vi "pyonpyon3.vi"() -> ()   [LabVIEW 2013]
uses:
  impl/pp3_CTL_SessionInfo.ctl
  impl/pp3_CTL_StateInfo.ctl
  impl/pp3_CTL_State.ctl
  impl/pp3_CTL_Trial.ctl
  impl/pp3_CTL_TrialType.ctl
  labolabo2/waveforms/WFTypes.ctl
  impl/pp2_CTL_SessionParamDynamic.ctl
  impl/pp2_CTL_DaqConfig.ctl
  <vilib>/userdefined/High Color/IMAQdx.ctl
  <vilib>/sound2/lvsound2.llb/Sound Output Task ID.ctl
  labolabo2/array/impl/NullArray_I.vi
  <vilib>/Utility/file.llb/Read From Spreadsheet File (string).vi
  labolabo2/array/impl/ArrayFirst_S.vi
panel:
  in  "Session List Hidden":u8[](array[numeric]) min=1 step=1
  out "concatenated string":string="OS Name:                   Microsoft Wi\rOS Version:                6.1.7601 Service Pack 1 Build 7601\rSystem Type:               x64-based PC\rTime Zone:                 (UTC+01:00) Amsterdam, Berli\rTotal Physical Memory:     7,657 MB"
  out "Info VI Revision":string="1221" caption="Rev #"
  out "Info VI Name":string="pyonpyon2.vi"
  out "Info Hostname":string="PCR6985-17"
  out "Session list display":string[][](table)
  in  "Trial Types Control":enum32{"Trial Types Control"}(tab)
  out "Trial Types File Path":path=path "E:/Data/SPP.Coulb1/trial types/FM2k4k_4k2k.pp2tt.tsv"
  in  "Save Trial Types":bool
  in  "Load Trial Types":bool
  out "Trial Types Valid":bool
  in  "Trial Types":T1[](array[typedef])=[{"Trial Type Number"=1, "Trial Type"=enum."GO", "Trial Weight"=1, "Shock (mA)"=-1.0, "Duration (ms)"=250.0, "Sound Type"=enum."04 FM Sweep", "Stim P1"=2000.0, "Stim P2"=4000.0, "Stim P3"=0.0, "Stim P4"=0.0, "DAQ Amplitude (V)"=0.25}, {"Trial Type Number"=2, "Trial Type"=enum."NOGO", "Trial Weight"=1, "Shock (mA)"=-1.0, "Duration (ms)"=250.0, "Sound Type"=enum."04 FM Sweep", "Stim P1"=4000.0, "Stim P2"=2000.0, "Stim P3"=0.0, "Stim P4"=0.0, "DAQ Amplitude (V)"=0.25}] {"DAQ Amplitude (V)" min=0.0 max=5.0 format="%_6g"; "Shock (mA)" min=-1.0 max=5.0; "Trial Weight" step=1; "Duration (ms)" min=0.0 max=1.0; "Trial Type Number" min=1 max=256 step=1}
  in  "Session List Control":enum32{"Session List Control"}(tab)
  out "Session List File Path":path
  in  "Load Session List":bool
  in  "Save Session List":bool
  in  "Generate Session List":bool
  in  "Total Trials":i32=60 min=3 max=122 step=1
  in  "Pseudo-Gellerman\nStart":i32=2 min=0 max=3 step=1
  out "Session List Valid":bool
  in  "Daq config":T4={"Sound AO"="Dev3/ao0", "Shock intesity AO"="Dev3/ao1", "Code_LED DO"="Dev3/port0", "Switch DI"="Dev3/port2/line0", "Webcam"="cam9", "Sound AO task"="", "Sound card task"=0, "Shock intensity AO task"="", "Code_LED DO task"="", "Switch DI task"="", "AO <=> Sound card"=FALSE, "Sound card"=0, "sample rate"=100000.0, "Variable shock"=TRUE, "Webcam on"=TRUE, "Tone gate PFI"="/Dev3/PFI0", "Waveform memo"={"t0"=timestamp(0 s since 1904-01-01), "dt"=1.0, "Y"=[]}, "First time"=FALSE} {"sample rate" min=8000.0; "Sound card task" format="%.0x"}
  out "Image":T7(plugin-control)
  in  "Session param (dynamic)":T8={"Def M shock (mA)"=700.0, "Def F shock (mA)"=140.0, "Def M shock +/-"=4, "Def F shock +/-"=4} {"Def F shock +/-" min=0 step=1; "Def M shock +/-" min=0 step=1}
  in  "stop":bool
  in  "Pause":bool
  out "State info":T9={"Curr  tr"=6, "Curr (ms)"=314431, "Cum (ms)"=205111, "Run loop diff"=6, "Tone countdown (ms)"=999999, "Countdown (ms)"=-1, "Curr State"=enum."15 Done", "Prev State"=enum."14 Intertrial Interval", "Rw"=FALSE, "Sw"=TRUE, "Tone\nGate"=FALSE, "Punish"=FALSE, "Current DAQ DO Int"=0, "Current Loaded Trial"={"Trial Type Number"=2, "Trial Type"=enum."NOGO", "Trial Weight"=1, "Shock (mA)"=0.0, "Duration (ms)"=250.0, "Sound Type"=enum."04 FM Sweep", "Stim P1"=4000.0, "Stim P2"=2000.0, "Stim P3"=0.0, "Stim P4"=0.0, "DAQ Amplitude (V)"=0.25}, "Next Trial (for display purposes)"={"Trial Type Number"=1, "Trial Type"=enum."GO", "Trial Weight"=1, "Shock (mA)"=-1.0, "Duration (ms)"=250.0, "Sound Type"=enum."04 FM Sweep", "Stim P1"=2000.0, "Stim P2"=4000.0, "Stim P3"=0.0, "Stim P4"=0.0, "DAQ Amplitude (V)"=0.25}, "Total trials memo"=6, "State start cum memo (ms)"=190105, "Last dur jump time memo (ms)"=0, "Last dur shock time memo (ms)"=0, "Tone repeat memo (ms)"=0, "Webcam on"=TRUE, "Webcam recording"=FALSE, "State update flag"=FALSE, "Last loaded shock voltage"=0.0, "Vid upd"=enum."0"} {"Current DAQ DO Int" format="%016b"; "Next Trial (for display purposes)"."DAQ Amplitude (V)" min=0.0 max=5.0 format="%_6g"; "Next Trial (for display purposes)"."Shock (mA)" min=-1.0 max=5.0; "Next Trial (for display purposes)"."Trial Weight" step=1; "Next Trial (for display purposes)"."Duration (ms)" min=0.0 max=1.0; "Next Trial (for display purposes)"."Trial Type Number" min=1 max=256 step=1; "Current Loaded Trial"."DAQ Amplitude (V)" min=0.0 max=5.0 format="%_6g"; "Current Loaded Trial"."Shock (mA)" min=-1.0 max=5.0; "Current Loaded Trial"."Trial Weight" step=1; "Current Loaded Trial"."Duration (ms)" min=0.0 max=1.0; "Current Loaded Trial"."Trial Type Number" min=1 max=256 step=1}
  in  "Session parameters":T11={"Log File Directory Root"=path "E:/Data/SPP.Coulb1", "Habit tr0 (s)"=180, "ITI max\n(s)"=24, "ITI min\n(s)"=14, "Tone repeat (ms)"=0, "Jump time\n(s)"=4, "Subject Name"="SPP046", "Run"=FALSE, "Start trial"=0, "Stay \n(s)"=5, "Log File Directory"=path "E:/Data/SPP.Coulb1/Test/150117/130444", "Shock \ndur (s)"=6, "Pre click \n(V)"=0.1, "Click\ndel (s)"=1.0, "Reward CR"=FALSE} {"Click\ndel (s)" min=0.0 step=1.0; "Pre click \n(V)" min=0.0 max=1.0 step=1.0; "Shock \ndur (s)" min=0 step=1; "Stay \n(s)" min=0 step=1; "Start trial" step=1; "Jump time\n(s)" min=0 step=1; "Tone repeat (ms)" min=0 max=1000 step=1; "ITI min\n(s)" min=0 step=1; "ITI max\n(s)" min=0 step=1; "Habit tr0 (s)" min=0 step=1}
  out "Runtime Errors":errorcluster
  in  "Refresh":bool
  out "Session info":T12={"Total  Tr"=6, "G Tr"=3, "G Jump"=0, "G Jump%"=0.0, "N Tr"=3, "N Jump"=0, "N Jump%"=0.0, "T Tr"=0, "T Jump"=0, "T Jump%"=nan, "M shock dur (ms)"=59414.666666666664, "F shock dur (ms)"=0.0, "H latency (ms)"=0.0, "F latency (ms)"=0.0, "T jump latency (ms)"=0.0} {"T Jump%" format="%.3g"; "N Jump%" format="%.3g"; "G Jump%" format="%.3g"}
  # "Pyonpyon Labview  v3 \n(2015.10 KT)"
  # "Code"
  # "Type"
  # "Dur (ms)"
  # "P 1"
  # "P 2"
  # "P 3"
  # "P 4"
  # "Weight"
  # "Shock"
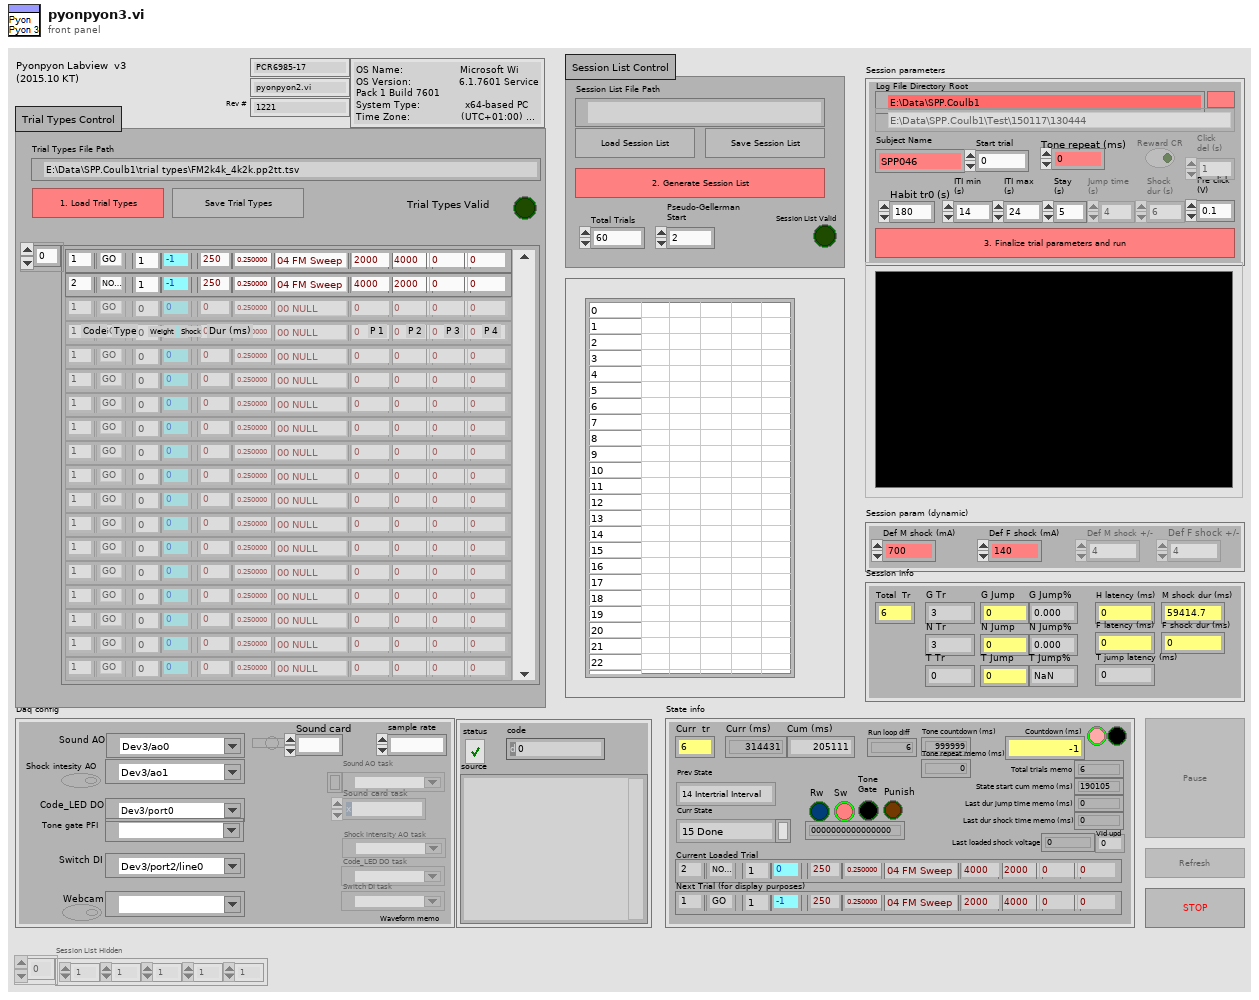
[diagram p1: front panel]
types:
  T1 = typedef "pp3_CTL_Trial.ctl" = cluster{"Trial Type Number":i16, "Trial Type":T2, "Trial Weight":u32, "Shock (mA)":dbl, "Duration (ms)":dbl, "Sound Type":T3, "Stim P1":dbl, "Stim P2":dbl, "Stim P3":dbl, "Stim P4":dbl, "DAQ Amplitude (V)":dbl}
  T2 = typedef "pp3_CTL_TrialType.ctl" = enum16{"OFF", "GO", "NOGO", "TEST"}
  T3 = typedef "WFTypes.ctl" = enum16{"00 NULL", "01 DC", "02 Noise", "03 Pure Tone", "04 FM Sweep"}
  T4 = typedef "pp2_CTL_DaqConfig.ctl" = cluster{"Sound AO":tag, "Shock intesity AO":tag, "Code_LED DO":tag, "Switch DI":tag, "Webcam":T5, "Sound AO task":refnum<k21>, "Sound card task":T6, "Shock intensity AO task":refnum<k21>, "Code_LED DO task":refnum<k21>, "Switch DI task":refnum<k21>, "AO <=> Sound card":bool, "Sound card":u32, "sample rate":dbl, "Variable shock":bool, "Webcam on":bool, "Tone gate PFI":tag, "Waveform memo":waveform(dbl), "First time":bool}
  T5 = typedef "IMAQdx.ctl" = refnum<k21>
  T6 = typedef "Sound Output Task ID.ctl" = u32
  T7 = typedef "IMAQ Image.ctl" = refnum<image>
  T8 = typedef "pp2_CTL_SessionParamDynamic.ctl" = cluster{"Def M shock (mA)":dbl, "Def F shock (mA)":dbl, "Def M shock +/-":i32, "Def F shock +/-":i32}
  T9 = typedef "pp3_CTL_StateInfo.ctl" = cluster{"Curr  tr":u16, "Curr (ms)":u32, "Cum (ms)":i64, "Run loop diff":i64, "Tone countdown (ms)":i64, "Countdown (ms)":i64, "Curr State":T10, "Prev State":T10, "Rw":bool, "Sw":bool, "Tone\nGate":bool, "Punish":bool, "Current DAQ DO Int":u16, "Current Loaded Trial":T1, "Next Trial (for display purposes)":T1, "Total trials memo":i64, "State start cum memo (ms)":i64, "Last dur jump time memo (ms)":i64, "Last dur shock time memo (ms)":i64, "Tone repeat memo (ms)":i64, "Webcam on":bool, "Webcam recording":bool, "State update flag":bool, "Last loaded shock voltage":dbl, "Vid upd":enum16{"0", "1", "2", "3", "4", "5", "6", "7", "8", "9"}}
  T10 = typedef "pp3_CTL_State.ctl" = enum8{"0 NULL", "1 Habituation", "2 (Load Trial)", "3 Stay Period", "4 Load Audio/Click Delay", "5 GO Trial", "6 GO Jumped", "7 GO Timeout", "8 NOGO Trial", "9 NOGO Jumped", "10 NOGO Timeout", "11 TEST Trial", "12 TEST Jumped", "13 TEST Timeout", "14 Intertrial Interval", "15 Done"}
  T11 = cluster{"Log File Directory Root":path, "Habit tr0 (s)":i32, "ITI max\n(s)":i32, "ITI min\n(s)":i32, "Tone repeat (ms)":i32, "Jump time\n(s)":i32, "Subject Name":string, "Run":bool, "Start trial":u16, "Stay \n(s)":i32, "Log File Directory":path, "Shock \ndur (s)":i32, "Pre click \n(V)":dbl, "Click\ndel (s)":dbl, "Reward CR":bool}
  T12 = typedef "pp3_CTL_SessionInfo.ctl" = cluster{"Total  Tr":u32, "G Tr":u32, "G Jump":u32, "G Jump%":dbl, "N Tr":u32, "N Jump":u32, "N Jump%":dbl, "T Tr":u32, "T Jump":u32, "T Jump%":dbl, "M shock dur (ms)":dbl, "F shock dur (ms)":dbl, "H latency (ms)":dbl, "F latency (ms)":dbl, "T jump latency (ms)":dbl}
  T13 = enum8{"Enabled", "Disabled", "Disabled and Grayed Out"}
  T14 = enum16{"open", "replace", "create", "open or create", "replace or create", "replace or create with confirmation"}
  T15 = typedef "imagedata.ctl" = cluster{"image type":i32, "image depth":i32, "image":u8[], "mask":u8[], "colors":u32[], "Rectangle":cluster{"left":i16, "top":i16, "right":i16, "bottom":i16}}
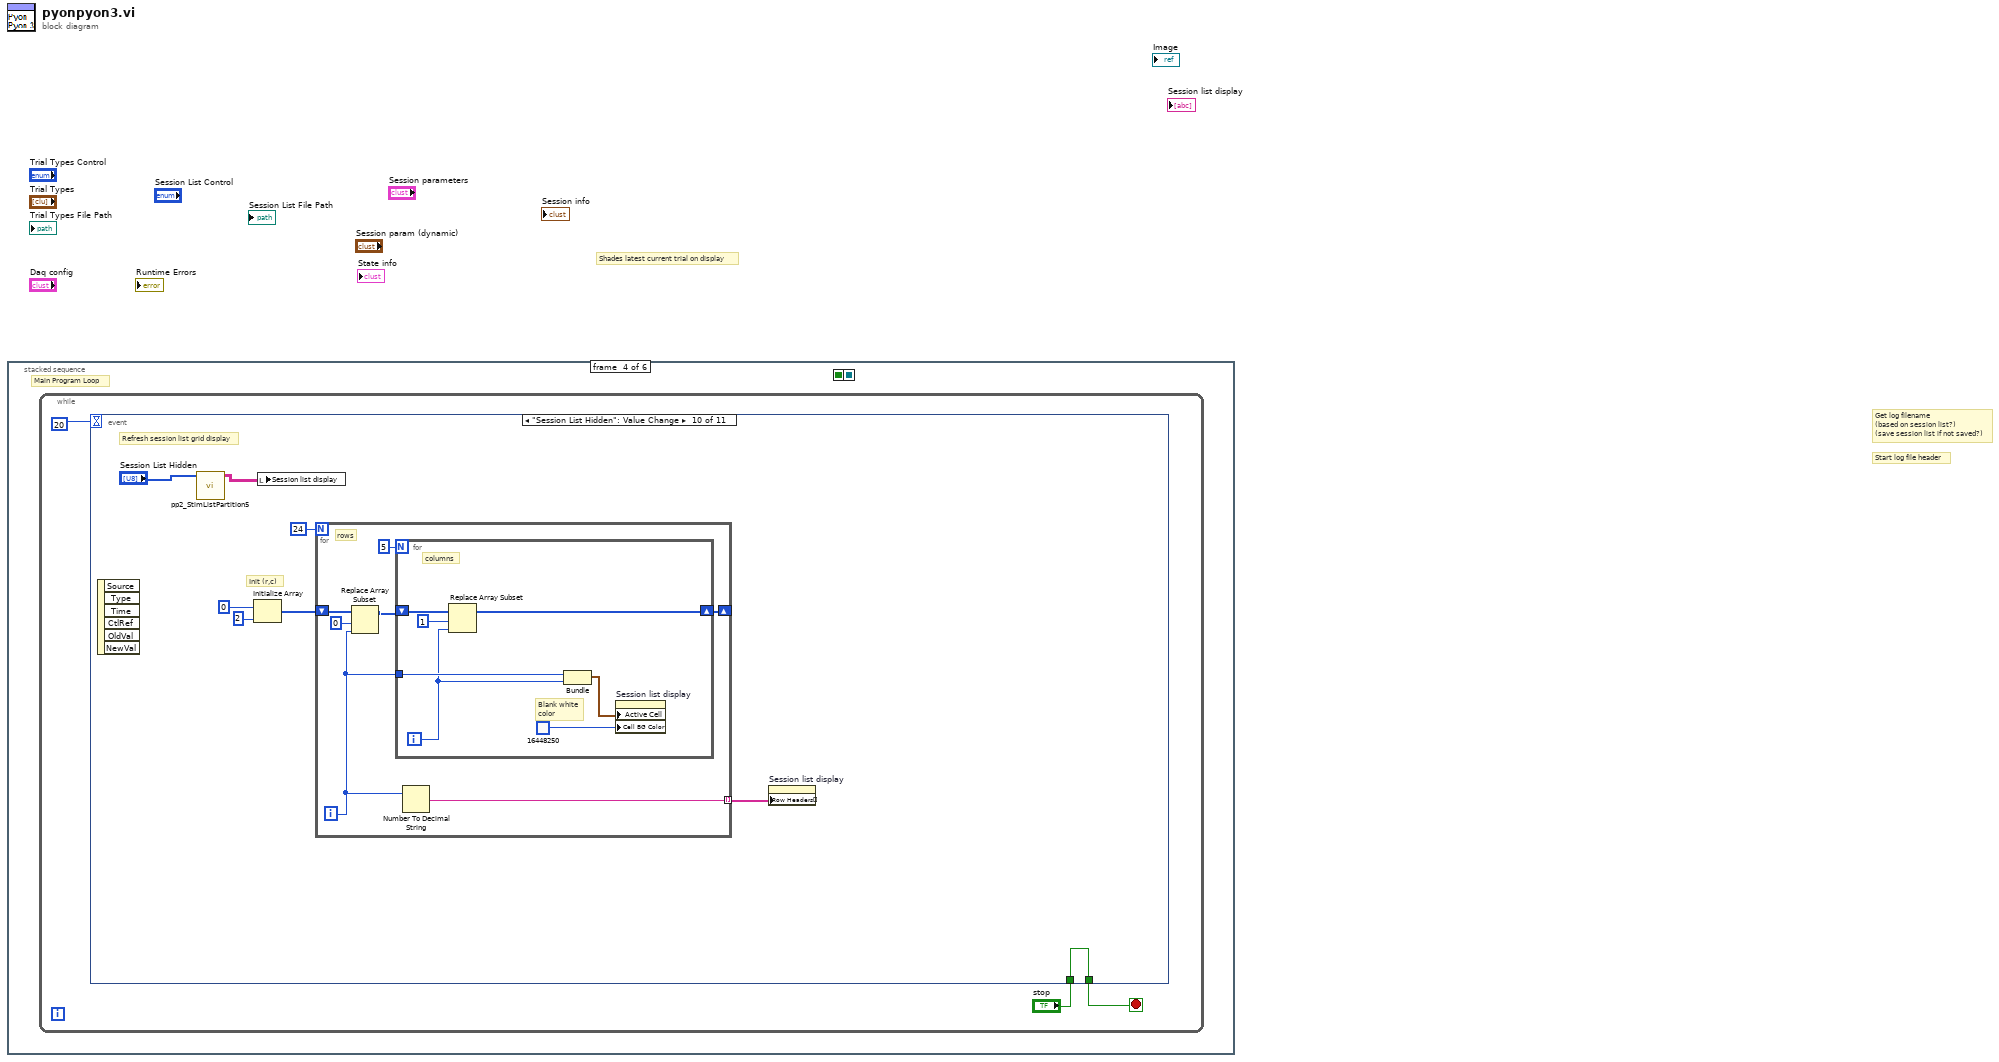
[diagram p0: block diagram]
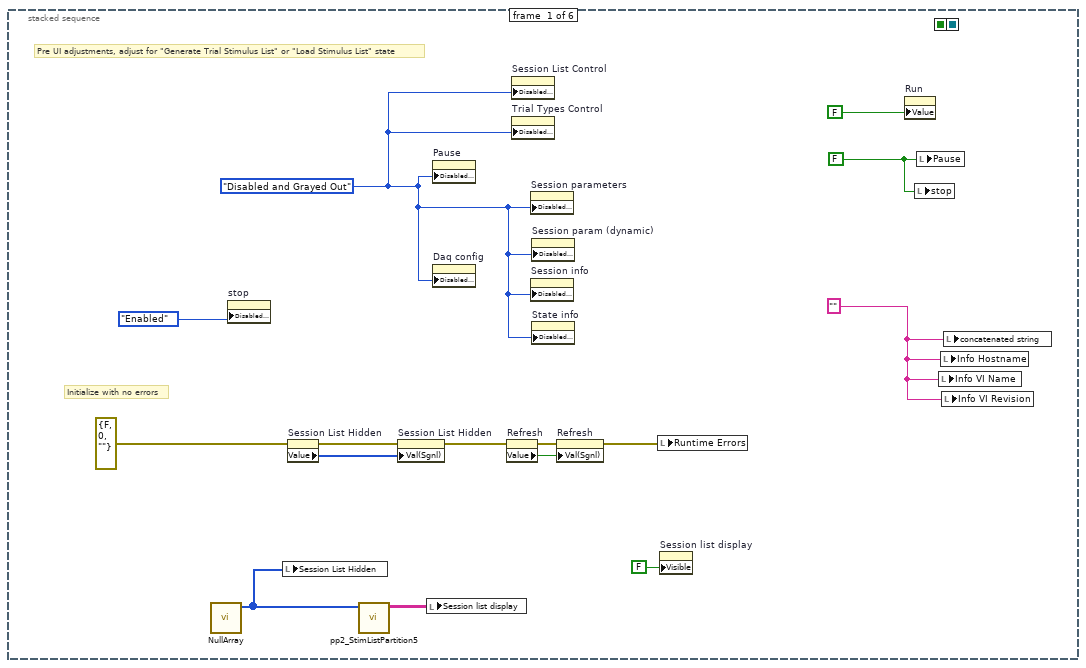
[diagram p2: hidden frame]
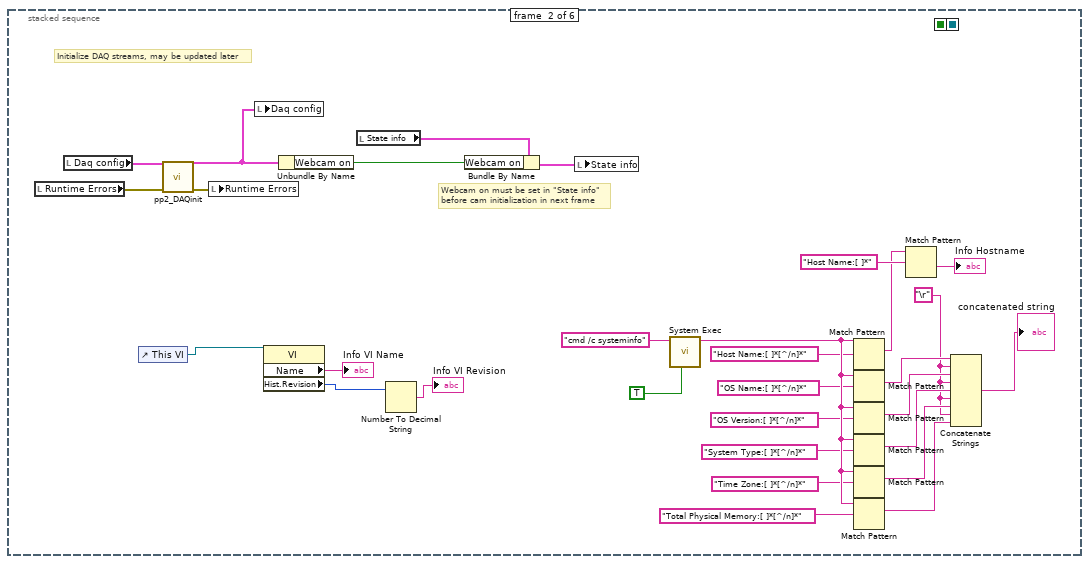
[diagram p3: hidden frame]
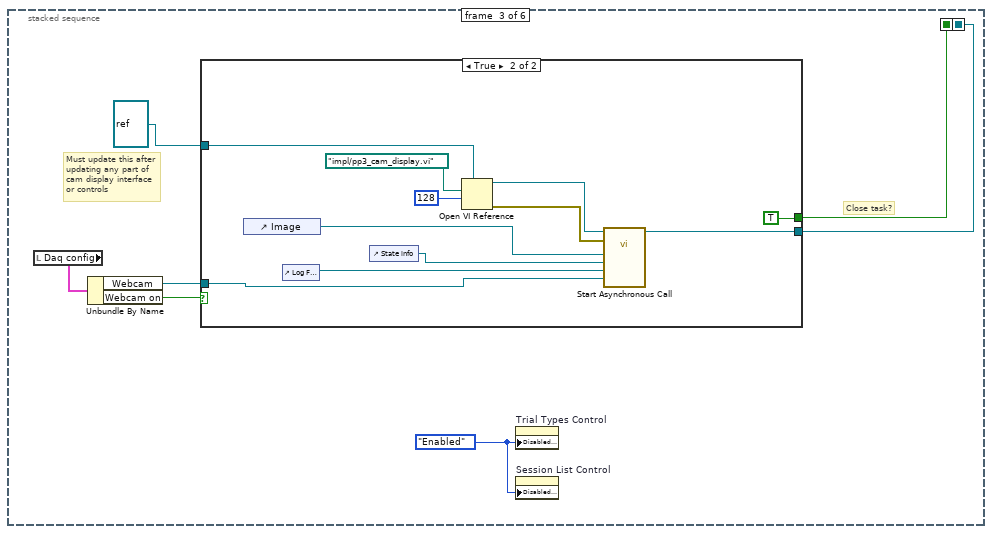
[diagram p4: hidden frame]
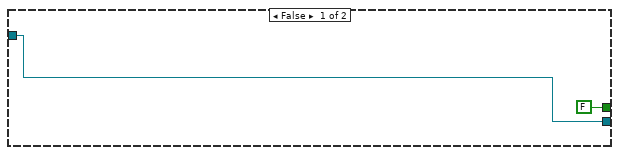
[diagram p5: hidden frame]
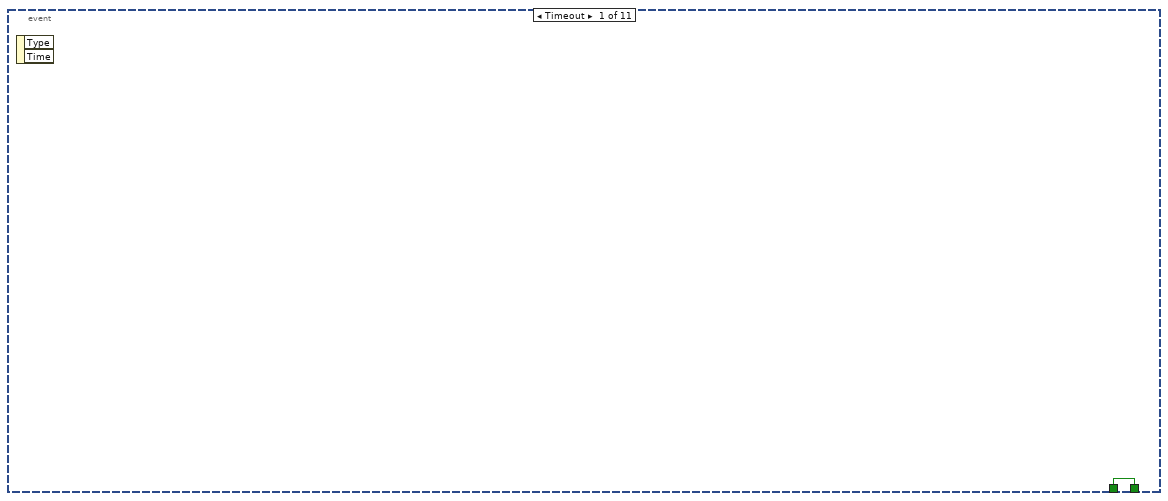
[diagram p6: hidden frame]
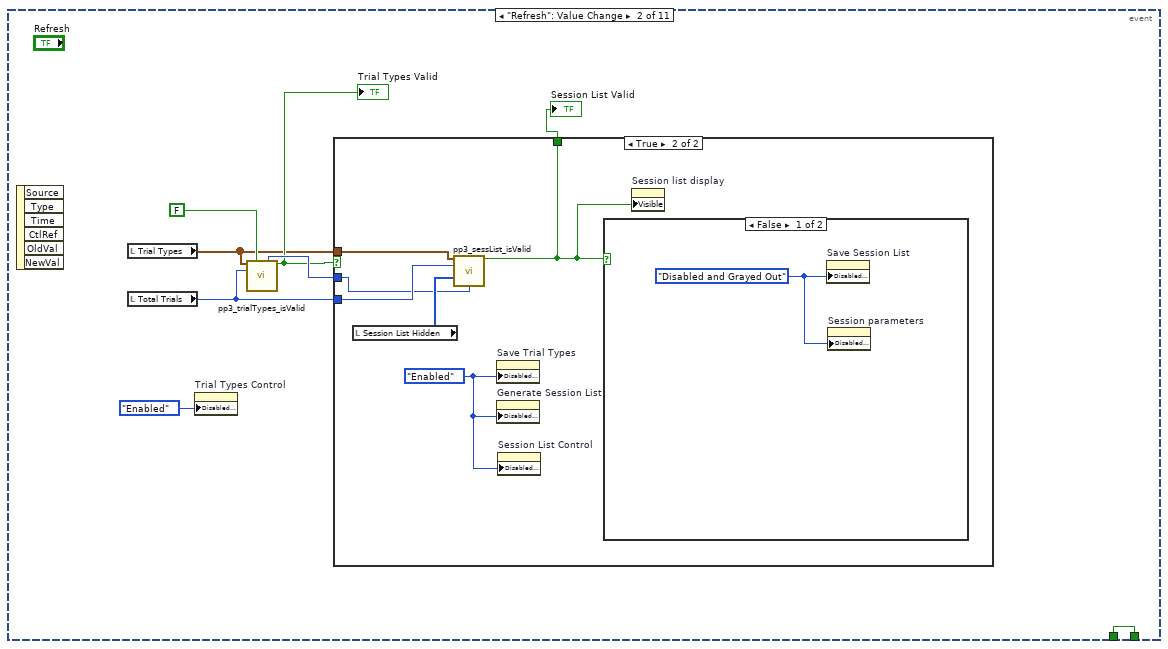
[diagram p7: hidden frame]
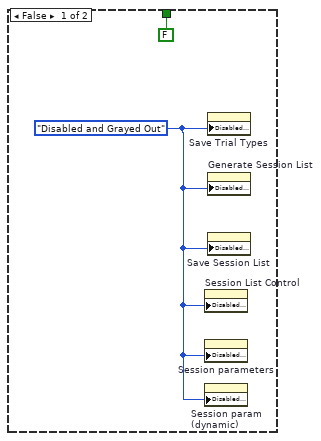
[diagram p8: hidden frame]
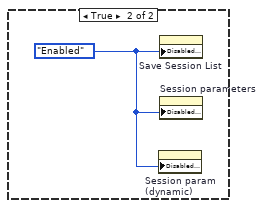
[diagram p9: hidden frame]
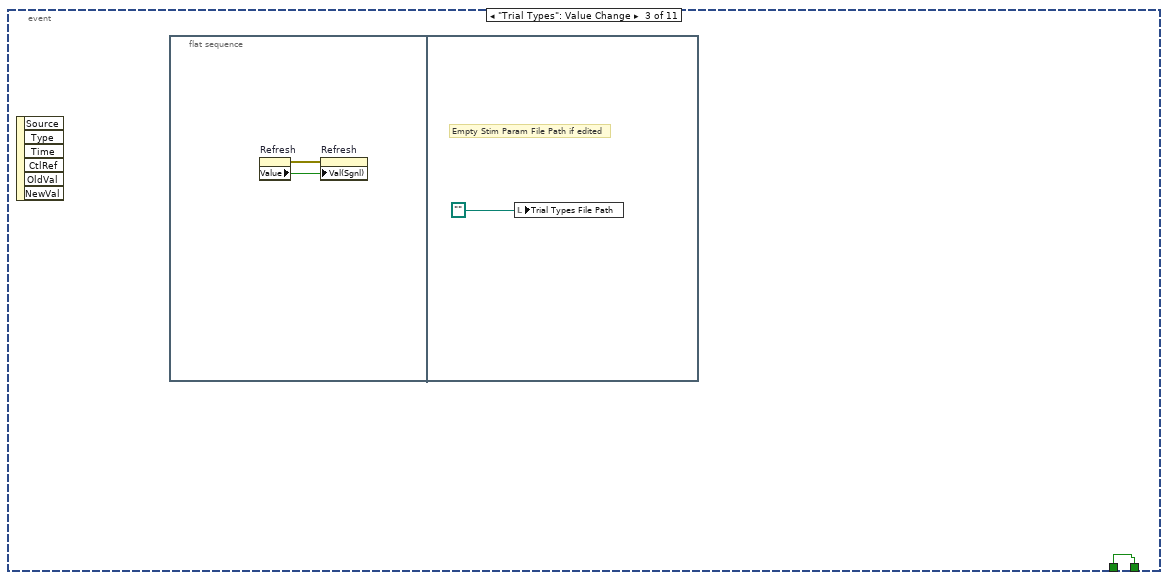
[diagram p10: hidden frame]
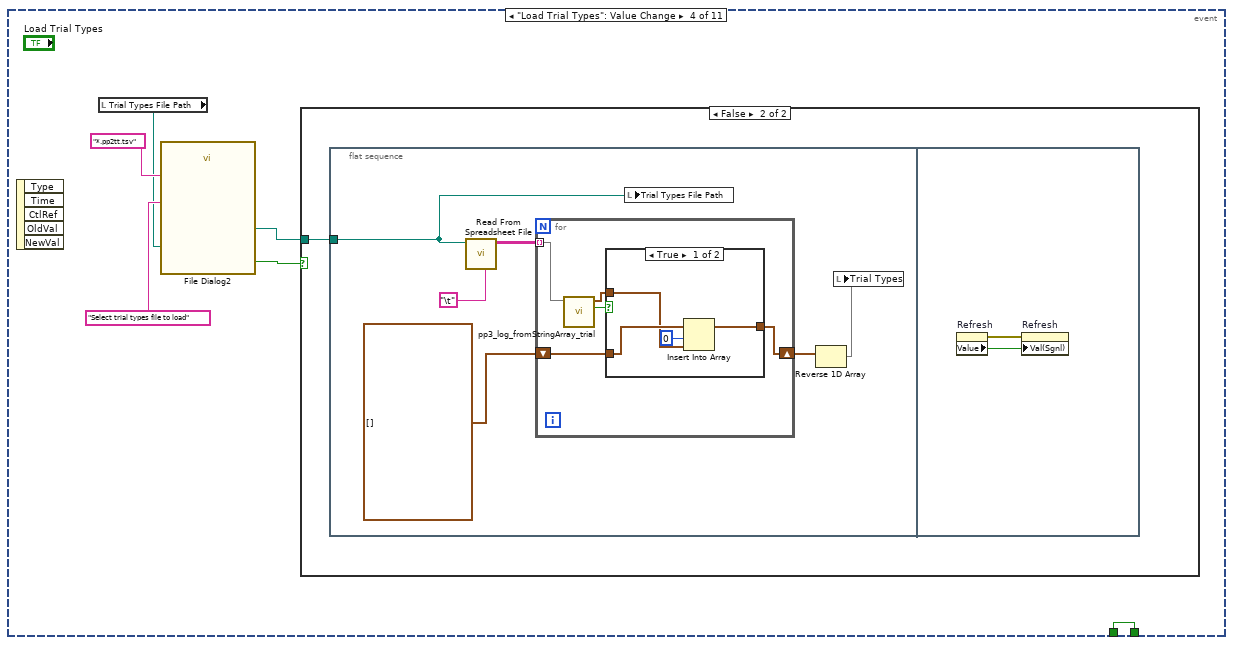
[diagram p11: hidden frame]
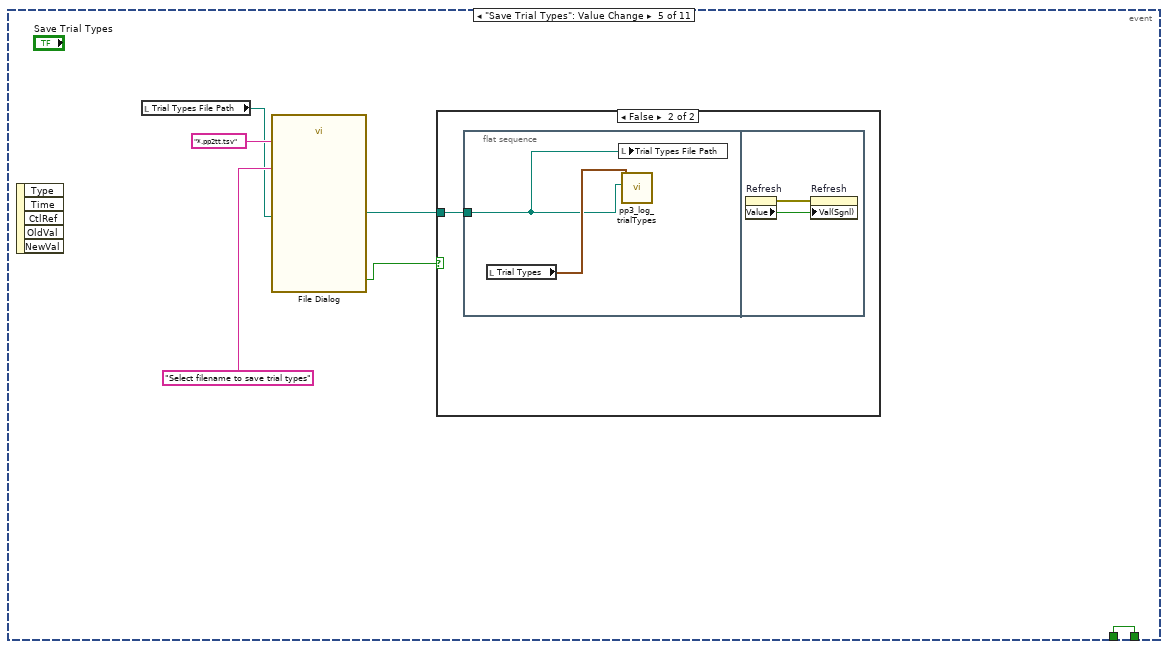
[diagram p14: hidden frame]
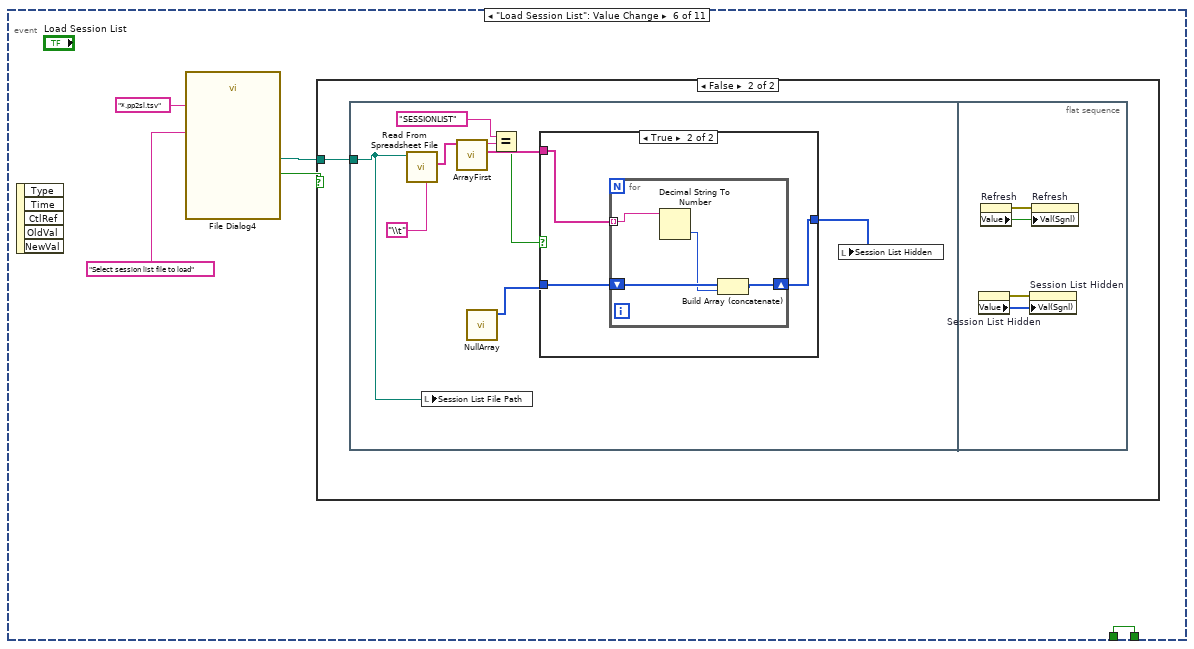
[diagram p16: hidden frame]
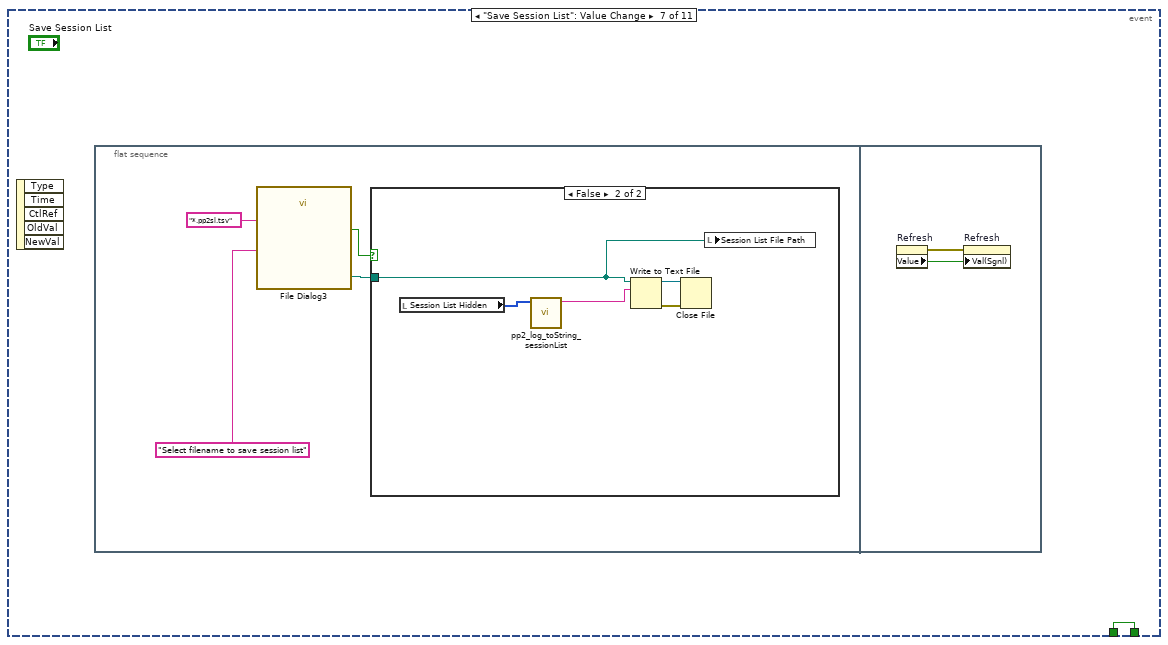
[diagram p19: hidden frame]
diagram:
  # "Shades latest current trial on display"
  # "Start log file header"
  # "Get log filename\n(based on session list?)\n(save session list if not saved?)"
  n1 = stacked-sequence {
    seq-local: [_ _ w49 _ _ _] -> [_ _ _ _ w714 _]
    seq-local: [_ _ w48 _ _ _] -> [_ _ _ _ w711 _]
    frame #0 {
      w2 = "" ("concatenated string")
      w15 = FALSE
      w1 = T13."Disabled and Grayed Out" ("Disabled")
      # "Initialize with no errors"
      # "Pre UI adjustments, adjust for \"Generate Trial Stimulus List\" or \"Load Stimulus List\" state"
      n2 = call-poly "NullArray.vi"() -> ("Null Array"=w6:i32[])  [unwired: 11 in]
      n3 = property on="stop" class="Bool (strict)"("DisabledEnum"=T13."Enabled" ("Disabled")) -> ()  [unwired: 2 in, 2 out]
      n4 = local write "Session List Hidden"(w6) -> ()
      n5 = property on="Session List Hidden" class="Arr (strict)"(error in=errorcluster {"status"=FALSE, "code"=0, "source"=""} ("error in (no error)")) -> (error out=w12:errorcluster, "Value"=w11:u8[])  [unwired: 1 in, 1 out]
      n6 = call "pp2_StimListPartition5.vi"("Session List (Hidden variable)"=w6) -> ("Session list display"=w5:string[][])  [unwired: 9 in]
      n7 = property on="Session List Hidden" class="Arr (strict)"(error in=w12, "Val(Sgnl)"=w11) -> (error out=w9:errorcluster)  [unwired: 1 in, 1 out]
      n8 = local write "Session list display"(w5) -> ()
      n9 = property on="Pause" class="Bool (strict)"("DisabledEnum"=w1) -> ()  [unwired: 2 in, 2 out]
      n10 = property on="Daq config" class="Clust (strict)"("DisabledEnum"=w1) -> ()  [unwired: 2 in, 2 out]
      n11 = property on="Refresh" class="Bool (strict)"(error in=w9) -> (error out=w8:errorcluster, "Value"=w10:bool)  [unwired: 1 in, 1 out]
      n12 = property on="Session List Control" class="TabCtl (strict)"("DisabledEnum"=w1) -> ()  [unwired: 2 in, 2 out]
      n13 = property on="Trial Types Control" class="TabCtl (strict)"("DisabledEnum"=w1) -> ()  [unwired: 2 in, 2 out]
      n14 = property on="Session parameters" class="Clust (strict)"("DisabledEnum"=w1) -> ()  [unwired: 2 in, 2 out]
      n15 = property on="Session info" class="Clust (strict)"("DisabledEnum"=w1) -> ()  [unwired: 2 in, 2 out]
      n16 = property on="Session param (dynamic)" class="Clust (strict)"("DisabledEnum"=w1) -> ()  [unwired: 2 in, 2 out]
      n17 = property on="State info" class="Clust (strict)"("DisabledEnum"=w1) -> ()  [unwired: 2 in, 2 out]
      n18 = property on="Refresh" class="Bool (strict)"(error in=w8, "Val(Sgnl)"=w10) -> (error out=w7:errorcluster)  [unwired: 1 in, 1 out]
      n19 = local write "Runtime Errors"(w7) -> ()
      n20 = property on="Session list display" class="Tbl (strict)"("Visible"=FALSE) -> ()  [unwired: 2 in, 2 out]
      n21 = property on="Run" class="Bool (strict)"("Value"=FALSE) -> ()  [unwired: 2 in, 2 out]
      n22 = local write "stop"(w15) -> ()
      n23 = local write "Pause"(w15) -> ()
      n24 = local write "Info VI Name"(w2) -> ()
      n25 = local write "Info Hostname"(w2) -> ()
      n26 = local write "Info VI Revision"(w2) -> ()
      n27 = local write "concatenated string"(w2) -> ()
    }
    frame #1 {
      w24 = "\r"
      # "Webcam on must be set in \"State info\"\nbefore cam initialization in next frame"
      # "Initialize DAQ streams, may be updated later"
      n28 = local read "Runtime Errors"() -> (w40:errorcluster)
      n29 = local read "Daq config"() -> (w45:T4)
      n30 = control-ref of="This VI"() -> (w38:refnum<vi>)
      n31 = call "pp2_DAQinit.vi"("error in (no error)"=w40, "Daq config in"=w45) -> ("error out"=w39:errorcluster, "Daq config out"=w44:T4)  [unwired: 8 in]
      n32 = local write "Runtime Errors"(w39) -> ()
      n33 = local write "Daq config"(w44) -> ()
      n34 = property class="VI"(reference=w38) -> ("Name"=→"Info VI Name":string, "Hist.Revision"=w31:u32)  [unwired: 1 in, 2 out]
      n35 = Unbundle By Name(w44) -> ("Webcam on"=w42:bool)
      n36 = local read "State info"() -> (w43:T9)
      n37 = Number To Decimal String(number=w31) -> (decimal integer string=→"Info VI Revision":string)  [unwired: 1 in]
      n38 = Bundle By Name(cluster=w43, "Webcam on"=w42) -> (w41:T9)
      n39 = local write "State info"(w41) -> ()
      n40 = call <vilib>:"System Exec.vi"("run minimized? (F)"=TRUE, "command line"="cmd /c systeminfo") -> ("standard output"=w23:string)  [unwired: 6 in, 3 out]
      n41 = Match Pattern(string=w23, regular expression="Host Name:[ ]*[^/n]*") -> (match substring=w16:string)  [unwired: 1 in, 3 out]
      n42 = Match Pattern(string=w23, regular expression="OS Name:[ ]*[^/n]*") -> (match substring=w30:string)  [unwired: 1 in, 3 out]
      n43 = Match Pattern(string=w23, regular expression="OS Version:[ ]*[^/n]*") -> (match substring=w29:string)  [unwired: 1 in, 3 out]
      n44 = Match Pattern(string=w23, regular expression="System Type:[ ]*[^/n]*") -> (match substring=w28:string)  [unwired: 1 in, 3 out]
      n45 = Match Pattern(string=w23, regular expression="Time Zone:[ ]*[^/n]*") -> (match substring=w27:string)  [unwired: 1 in, 3 out]
      n46 = Match Pattern(string=w23, regular expression="Total Physical Memory:[ ]*[^/n]*") -> (match substring=w26:string)  [unwired: 1 in, 3 out]
      n47 = Match Pattern(string=w16, regular expression="Host Name:[ ]*") -> (after substring=→"Info Hostname":string)  [unwired: 1 in, 3 out]
      n48 = Concatenate Strings(w30, w24, w29, w24, w28, w24, w27, w24, w26) -> (→"concatenated string":string)
    }
    frame #2 {
      w47 = T13."Enabled" ("Disabled")
      # "Close task?"
      # "Must update this after\nupdating any part of\ncam display interface\nor controls"
      n49 = local read "Daq config"() -> (w51:T4)
      n50 = Unbundle By Name(w51) -> ("Webcam"=w52:T5, "Webcam on"=w50:bool)
      n51 = case shown="True" w50 {
        tunnel: w52 -> [_ w56]
        tunnel: [w54 w55] -> w49
        tunnel: refnum<vi> refnum ("type specifier VI Refnum (for type only)") -> [w54 w63]
        tunnel: [FALSE TRUE] -> w48
        frame False {
        }
        frame True {
          n52 = control-ref of="Image"() -> (w59:refnum<vi>)
          n53 = control-ref of="Log File Directory"() -> (w57:refnum<vi>)
          n54 = control-ref of="State info"() -> (w58:refnum<vi>)
          n55 = Open VI Reference(type specifier VI Refnum (for type only)=w63, vi path=path "impl/pp3_cam_display.vi", options=128) -> (vi reference=w60:refnum<vi>, error out=w61:errorcluster)  [unwired: 3 in]
          n56 = call-by-ref "Start Asynchronous Call"(reference=w60, error in=w61, "Camera"=w56, "Log File Directory"=w57, "State info Refnum"=w58, "Image Ctl Refnum"=w59) -> (reference out=w55:refnum<vi>)  [unwired: 8 in, 1 out]
        }
      }
      n57 = property on="Trial Types Control" class="TabCtl (strict)"("DisabledEnum"=w47) -> ()  [unwired: 2 in, 2 out]
      n58 = property on="Session List Control" class="TabCtl (strict)"("DisabledEnum"=w47) -> ()  [unwired: 2 in, 2 out]
    }
    frame #3 {
      # "Main Program Loop"
      n59 = while {
        stop <- w68 stop-if-true
        n60 = event shown="[9] \"Session List Hidden\": Value Change" {
          selector: _ -> [_ _ _ _ _ _ _ _ _ _ _]
          dyn-events: _ -> [_ _ _ _ _ _ _ _ _ _ _]
          timeout: u32 20 ("milliseconds to wait") -> [_ _ _ _ _ _ _ _ _ _ _]
          tunnel: [w69 w70 w88 w97 w122 w132 w155 w167 w179 w183 w205] -> w68
          tunnel: "stop" -> [w69 w70 w88 w97 w122 w132 w155 w167 w179 w183 _]
          event Timeout {
            n61 = event-data() -> ()  [unwired: 1 in, 2 out]
          }
          event "Refresh": Value Change {
            n62 = event-data() -> ()  [unwired: 1 in, 6 out]
            n63 = local read "Trial Types"() -> (w73:T1[])
            n64 = local read "Total Trials"() -> (w76:i32)
            n65 = property on="Trial Types Control" class="TabCtl (strict)"("DisabledEnum"=T13."Enabled" ("Disabled")) -> ()  [unwired: 2 in, 2 out]
            n66 = call "pp3_trialTypes_isValid.vi"("Trial Types In"=w73, "Throw Error"=FALSE, "Total Trials"=w76) -> ("Trial Replication Factor"=w77:i32, "Paradigm Valid?"=w74:bool)  [unwired: 7 in, 4 out]
            "Trial Types Valid" <- w74
            n67 = case shown="True" w74 {
              tunnel: w77 -> [_ w82]
              tunnel: w76 -> [_ w85]
              tunnel: w73 -> [_ w84]
              tunnel: [FALSE ("Session List Valid?") w80] -> w72
              frame False {
                w78 = T13."Disabled and Grayed Out" ("Disabled")
                n68 = property on="Session List Control" class="TabCtl (strict)"("DisabledEnum"=w78) -> ()  [unwired: 2 in, 2 out]
                n69 = property on="Session parameters" class="Clust (strict)"("DisabledEnum"=w78) -> ()  [unwired: 2 in, 2 out]
                n70 = property on="Session param (dynamic)" class="Clust (strict)"("DisabledEnum"=w78) -> ()  [unwired: 2 in, 2 out]
                n71 = property on="Save Trial Types" class="Bool"("DisabledEnum"=w78) -> ()  [unwired: 2 in, 2 out]
                n72 = property on="Generate Session List" class="Bool"("DisabledEnum"=w78) -> ()  [unwired: 2 in, 2 out]
                n73 = property on="Save Session List" class="Bool"("DisabledEnum"=w78) -> ()  [unwired: 2 in, 2 out]
              }
              frame True {
                w81 = T13."Enabled" ("Disabled")
                n74 = local read "Session List Hidden"() -> (w83:u8[])
                n75 = call "pp3_sessList_isValid.vi"("Trial Types In"=w84, "Total Trials"=w85, "Session List"=w83, "Trial Replication Factor"=w82) -> ("Session List Valid?"=w80:bool)  [unwired: 11 in]
                n76 = property on="Save Trial Types" class="Bool"("DisabledEnum"=w81) -> ()  [unwired: 2 in, 2 out]
                n77 = property on="Generate Session List" class="Bool"("DisabledEnum"=w81) -> ()  [unwired: 2 in, 2 out]
                n78 = property on="Session List Control" class="TabCtl (strict)"("DisabledEnum"=w81) -> ()  [unwired: 2 in, 2 out]
                n79 = case shown="False" w80 {
                  frame False {
                    w86 = T13."Disabled and Grayed Out" ("Disabled")
                    n80 = property on="Save Session List" class="Bool"("DisabledEnum"=w86) -> ()  [unwired: 2 in, 2 out]
                    n81 = property on="Session parameters" class="Clust (strict)"("DisabledEnum"=w86) -> ()  [unwired: 2 in, 2 out]
                  }
                  frame True {
                    w87 = T13."Enabled" ("Disabled")
                    n82 = property on="Session param (dynamic)" class="Clust (strict)"("DisabledEnum"=w87) -> ()  [unwired: 2 in, 2 out]
                    n83 = property on="Save Session List" class="Bool"("DisabledEnum"=w87) -> ()  [unwired: 2 in, 2 out]
                    n84 = property on="Session parameters" class="Clust (strict)"("DisabledEnum"=w87) -> ()  [unwired: 2 in, 2 out]
                  }
                }
                n85 = property on="Session list display" class="Tbl (strict)"("Visible"=w80) -> ()  [unwired: 2 in, 2 out]
              }
            }
            "Session List Valid" <- w72
          }
          event "Trial Types": Value Change {
            n86 = event-data() -> ()  [unwired: 1 in, 6 out]
            n87 = flat-sequence {
              frame #0 {
                n88 = property on="Refresh" class="Bool (strict)"() -> (error out=w90:errorcluster, "Value"=w89:bool)  [unwired: 2 in, 1 out]
                n89 = property on="Refresh" class="Bool (strict)"(error in=w90, "Val(Sgnl)"=w89) -> ()  [unwired: 1 in, 2 out]
              }
              frame #1 {
                # "Empty Stim Param File Path if edited"
                n90 = local write "Trial Types File Path"(path "") -> ()
              }
            }
          }
          event "Load Trial Types": Value Change {
            n91 = event-data() -> ()  [unwired: 1 in, 5 out]
            n92 = local read "Trial Types File Path"() -> (w92:path)
            n93 = call "File Dialog2"("start path"=w92, "prompt"="Select trial types file to load", "pattern (all files)"="*.pp2tt.tsv") -> ("selected path"=w94:path, "cancelled"=w93:bool)  [unwired: 9 in, 2 out]
            n94 = case shown="False" w93 {
              tunnel: w94 -> [_ w98]
              frame True {
              }
              frame False {
                n95 = flat-sequence {
                  tunnel: w98 -> [w100]
                  frame #0 {
                    n96 = call-poly <vilib>:"Read From Spreadsheet File.vi"("delimiter (\\t)"="\t" ("delimiter (\\t)"), "file path (dialog if empty)"=w100) -> ("all rows"=w104:string[][])  [unwired: 5 in, 4 out]
                    n97 = for {
                      tunnel: w104 -> [w108] mode=indexing
                      shift-right: [w106] -> w102
                      shift-left: T1[] [] -> [w107]
                      n98 = call "pp3_log_fromStringArray_trial.vi"("Input string array"=w108) -> ("Was TRIAL?"=w105:bool, "Trial in"=w109:T1)  [unwired: 7 in]
                      n99 = case shown="True" w105 {
                        tunnel: w109 -> [w112 _]
                        tunnel: w107 -> [w113 w114]
                        tunnel: [w110 w114] -> w106
                        frame True {
                          n100 = Insert Into Array(array=w113, index=0, new element=w112) -> (w110:T1[])
                        }
                        frame False {
                        }
                      }
                    }
                    n101 = local write "Trial Types File Path"(w100) -> ()
                    n102 = Reverse 1D Array(array=w102) -> (reversed array=w101:T1[])
                    n103 = local write "Trial Types"(w101) -> ()
                  }
                  frame #1 {
                    n104 = property on="Refresh" class="Bool (strict)"() -> (error out=w116:errorcluster, "Value"=w115:bool)  [unwired: 2 in, 1 out]
                    n105 = property on="Refresh" class="Bool (strict)"(error in=w116, "Val(Sgnl)"=w115) -> ()  [unwired: 1 in, 2 out]
                  }
                }
              }
            }
          }
          event "Save Trial Types": Value Change {
            n106 = event-data() -> ()  [unwired: 1 in, 5 out]
            n107 = local read "Trial Types File Path"() -> (w118:path)
            n108 = call "File Dialog"("start path"=w118, "prompt"="Select filename to save trial types", "pattern (all files)"="*.pp2tt.tsv") -> ("selected path"=w119:path, "cancelled"=w117:bool)  [unwired: 9 in, 2 out]
            n109 = case shown="False" w117 {
              tunnel: w119 -> [_ w123]
              frame True {
              }
              frame False {
                n110 = flat-sequence {
                  tunnel: w123 -> [w124]
                  frame #0 {
                    n111 = local read "Trial Types"() -> (w125:T1[])
                    n112 = local write "Trial Types File Path"(w124) -> ()
                    n113 = call "pp3_log_trialTypes.vi"("Trial Types File Path"=w124, "Trial Types"=w125) -> ()  [unwired: 10 in]
                  }
                  frame #1 {
                    n114 = property on="Refresh" class="Bool (strict)"() -> (error out=w126:errorcluster, "Value"=w127:bool)  [unwired: 2 in, 1 out]
                    n115 = property on="Refresh" class="Bool (strict)"(error in=w126, "Val(Sgnl)"=w127) -> ()  [unwired: 1 in, 2 out]
                  }
                }
              }
            }
          }
          event "Load Session List": Value Change {
            n116 = event-data() -> ()  [unwired: 1 in, 5 out]
            n117 = call "File Dialog4"("prompt"="Select session list file to load", "pattern (all files)"="*.pp2sl.tsv") -> ("selected path"=w129:path, "cancelled"=w128:bool)  [unwired: 10 in, 2 out]
            n118 = case shown="False" w128 {
              tunnel: w129 -> [_ w133]
              frame True {
              }
              frame False {
                n119 = flat-sequence {
                  tunnel: w133 -> [w137]
                  frame #0 {
                    n120 = call-poly <vilib>:"Read From Spreadsheet File.vi"("delimiter (\\t)"="\\t" ("delimiter (\\t)"), "file path (dialog if empty)"=w137) -> ("first row"=w141:string[])  [unwired: 5 in, 4 out]
                    n121 = local write "Session List File Path"(w137) -> ()
                    n122 = call-poly "ArrayFirst.vi"("1D Array In"=w141) -> ("Rest of Array"=w138:string[], "First Element"=w140:string)  [unwired: 9 in]
                    n123 = call-poly "NullArray.vi"() -> ("Null Array"=w134:i32[])  [unwired: 11 in]
                    n124 = Equal?(x="SESSIONLIST", y=w140) -> (x = y?=w136:bool)
                    n125 = case shown="True" w136 {
                      tunnel: w138 -> [_ w146]
                      tunnel: [w143 w145] -> w135
                      tunnel: w134 -> [w143 w144]
                      frame False {
                      }
                      frame True {
                        n126 = for {
                          shift-right: [w150] -> w145
                          shift-left: w144 -> [w149]
                          tunnel: w146 -> [w148] mode=indexing
                          n127 = Decimal String To Number(string=w148) -> (number=w147:i32)  [unwired: 2 in, 1 out]
                          n128 = Build Array (concatenate)(w149, w147) -> (w150:i32[])
                        }
                      }
                    }
                    n129 = local write "Session List Hidden"(w135) -> ()
                  }
                  frame #1 {
                    n130 = property on="Session List Hidden" class="Arr (strict)"() -> (error out=w151:errorcluster, "Value"=w152:u8[])  [unwired: 2 in, 1 out]
                    n131 = property on="Refresh" class="Bool (strict)"() -> (error out=w154:errorcluster, "Value"=w153:bool)  [unwired: 2 in, 1 out]
                    n132 = property on="Session List Hidden" class="Arr (strict)"(error in=w151, "Val(Sgnl)"=w152) -> ()  [unwired: 1 in, 2 out]
                    n133 = property on="Refresh" class="Bool (strict)"(error in=w154, "Val(Sgnl)"=w153) -> ()  [unwired: 1 in, 2 out]
                  }
                }
              }
            }
          }
          event "Save Session List": Value Change {
            n134 = event-data() -> ()  [unwired: 1 in, 5 out]
            n135 = flat-sequence {
              frame #0 {
                n136 = call "File Dialog3"("prompt"="Select filename to save session list", "pattern (all files)"="*.pp2sl.tsv") -> ("selected path"=w159:path, "cancelled"=w158:bool)  [unwired: 10 in, 2 out]
                n137 = case shown="False" w158 {
                  tunnel: w159 -> [_ w162]
                  frame True {
                  }
                  frame False {
                    n138 = local read "Session List Hidden"() -> (w164:u8[])
                    n139 = call "pp2_log_toString_sessionList.vi"("Session List in"=w164) -> ("spreadsheet string"=w163:string)  [unwired: 10 in]
                    n140 = Write to Text File(file (use dialog)=w162, text=w163) -> (refnum out=w160:refnum<file>, error out=w161:errorcluster)  [unwired: 2 in, 1 out]
                    n141 = Close File(refnum=w160, error in=w161) -> ()  [unwired: 2 out]
                    n142 = local write "Session List File Path"(w162) -> ()
                  }
                }
              }
              frame #1 {
                n143 = property on="Refresh" class="Bool (strict)"() -> (error out=w166:errorcluster, "Value"=w165:bool)  [unwired: 2 in, 1 out]
                n144 = property on="Refresh" class="Bool (strict)"(error in=w166, "Val(Sgnl)"=w165) -> ()  [unwired: 1 in, 2 out]
              }
            }
          }
          event "Generate Session List": Value Change {
            n145 = event-data() -> ()  [unwired: 1 in, 5 out]
            n146 = flat-sequence {
              frame #0 {
                # "Empty file name if generating list"
                n147 = local read "Trial Types"() -> (w169:T1[])
                n148 = local read "Total Trials"() -> (w172:i32)
                n149 = local write "Session List File Path"(path "") -> ()
                n150 = call "pp3_sessList_createPseudoGellerman.vi"("Start Num"="Pseudo-Gellerman\nStart", "Total Trials"=w172, "Trial Types"=w169) -> ("Session List (Cannot Edit)"=w168:i32[])  [unwired: 7 in, 1 out]
                n151 = local write "Session List Hidden"(w168) -> ()
              }
              frame #1 {
                n152 = property on="Session List Hidden" class="Arr (strict)"() -> (error out=w174:errorcluster, "Value"=w173:u8[])  [unwired: 2 in, 1 out]
                n153 = property on="Session list display" class="Tbl (strict)"() -> (error out=w176:errorcluster, "Value"=w175:string[][])  [unwired: 2 in, 1 out]
                n154 = property on="Refresh" class="Bool (strict)"() -> (error out=w178:errorcluster, "Value"=w177:bool)  [unwired: 2 in, 1 out]
                n155 = property on="Session list display" class="Tbl (strict)"(error in=w176, "Val(Sgnl)"=w175) -> ()  [unwired: 1 in, 2 out]
                n156 = property on="Refresh" class="Bool (strict)"(error in=w178, "Val(Sgnl)"=w177) -> ()  [unwired: 1 in, 2 out]
                n157 = property on="Session List Hidden" class="Arr (strict)"(error in=w174, "Val(Sgnl)"=w173) -> ()  [unwired: 1 in, 2 out]
              }
            }
          }
          event "Total Trials": Value Change {
            n158 = event-data() -> ()  [unwired: 1 in, 6 out]
            n159 = flat-sequence {
              tunnel: "Total Trials" -> [_]
              frame #0 {
              }
              frame #1 {
                n160 = property on="Refresh" class="Bool (strict)"() -> (error out=w181:errorcluster, "Value"=w182:bool)  [unwired: 2 in, 1 out]
                n161 = property on="Refresh" class="Bool (strict)"(error in=w181, "Val(Sgnl)"=w182) -> ()  [unwired: 1 in, 2 out]
              }
            }
          }
          event "Session List Hidden": Value Change {
            # "Refresh session list grid display"
            # "Init (r,c)"
            n162 = event-data() -> ()  [unwired: 1 in, 6 out]
            n163 = call "pp2_StimListPartition5.vi"("Session List (Hidden variable)"="Session List Hidden") -> ("Session list display"=w189:string[][])  [unwired: 9 in]
            n164 = Initialize Array(0, 2 ("dimension size")) -> (w187:i32[])
            n165 = local write "Session list display"(w189) -> ()
            n166 = for {
              N: 24 -> [_]
              shift-right: [w193] -> _
              shift-left: w187 -> [w196]
              tunnel: [w191] -> w184 mode=indexing
              i -> [w192]
              # "rows"
              n167 = Replace Array Subset(array=w196, new element=w192, index=0) -> (w195:i32[])
              n168 = for {
                N: 5 -> [_]
                shift-right: [w202] -> w193
                shift-left: w195 -> [w203]
                tunnel: w192 -> [w201]
                i -> [w200]
                # "columns"
                # "Blank white\ncolor"
                n169 = Replace Array Subset(array=w203, new element=w200, index=1) -> (w202:i32[])
                n170 = Bundle(w201, w200) -> (w199:cluster{i32, i32})  [unwired: 1 in]
                n171 = property on="Session list display" class="Tbl (strict)"("Active Cell"=w199, "Cell BG Color"=u32 16448250) -> ()  [unwired: 2 in, 2 out]
              }
              n172 = Number To Decimal String(number=w192) -> (decimal integer string=w191:string)  [unwired: 1 in]
            }
            n173 = property on="Session list display" class="Tbl (strict)"("Row Headers[]"=w184) -> ()  [unwired: 2 in, 2 out]
          }
          event "Session parameters.Run": Value Change {
            # "Log Que"
            n174 = event-data() -> ()  [unwired: 1 in, 6 out]
            n175 = stacked-sequence {
              seq-local: [_ _ w277 _ _ _] -> [_ _ _ w322 _ _]
              seq-local: [_ _ _ w333 _ _] -> [_ _ _ _ w696 _]
              seq-local: [_ _ _ w320 _ _] -> [_ _ _ _ w695 _]
              tunnel: [_ _ _ w321 _ _] -> w205
              frame #0 {
                w206 = T13."Disabled" ("Disabled")
                w207 = T13."Disabled and Grayed Out" ("Disabled")
                # "Confirm if starting with nonzero trial"
                # "GUI Adjustments (pre)"
                n176 = local read "Session parameters"() -> (w208:T11)
                n177 = flat-sequence {
                  tunnel: w207 -> [w212]
                  frame #0 {
                    n178 = property on="Session List Control" class="TabCtl (strict)"("DisabledEnum"=w212) -> ()  [unwired: 2 in, 2 out]
                  }
                  frame #1 {
                    n179 = property on="Session list display" class="Tbl (strict)"("DisabledEnum"=T13."Disabled" ("Disabled")) -> ()  [unwired: 2 in, 2 out]
                  }
                }
                n180 = Unbundle By Name(w208) -> ("Start trial"=w209:u16)
                n181 = property on="Trial Types Control" class="TabCtl (strict)"("DisabledEnum"=w207) -> ()  [unwired: 2 in, 2 out]
                n182 = Not Equal To 0?(x=w209) -> (x != 0?=w210:bool)
                n183 = case shown="True" w210 {
                  tunnel: w209 -> [_ w217]
                  tunnel: w208 -> [_ w214]
                  frame False {
                  }
                  frame True {
                    n184 = Number To Decimal String(number=w217) -> (decimal integer string=w218:string)  [unwired: 1 in]
                    n185 = Concatenate Strings("Really start with nonzero trial?: " ("message"), w218) -> (w216:string)
                    n186 = Two Button Dialog(message=w216, 1:"No, start from zero" ("F button name (\"Cancel\")"), 2:"Yes" ("T button name (\"OK\")")) -> (T button?=w215:bool)
                    n187 = case shown="False" w215 {
                      tunnel: w214 -> [w224 _]
                      frame False {
                        n188 = Bundle By Name(cluster=w224, "Start trial"=u16 0) -> (w222:T11)
                        n189 = local write "Session parameters"(w222) -> ()
                      }
                      frame True {
                        # "Just proceed"
                      }
                    }
                  }
                }
                n190 = property on="Session parameters" class="Clust (strict)"("DisabledEnum"=w207) -> ()  [unwired: 2 in, 2 out]
                n191 = disable-structure shown="Disabled" {
                  frame Disabled {
                    n192 = property on="Pause" class="Bool (strict)"("DisabledEnum"=T13."Enabled" ("Disabled")) -> ()  [unwired: 2 in, 2 out]
                  }
                  frame Enabled {
                  }
                }
                n193 = property on="State info" class="Clust (strict)"("DisabledEnum"=w206) -> ()  [unwired: 2 in, 2 out]
                n194 = property on="Session info" class="Clust (strict)"("DisabledEnum"=w206) -> ()  [unwired: 2 in, 2 out]
              }
              frame #1 {
                # "ToDo... go through\nsequence for starting\nat trial !=0 for new\nlog, when state info is not\ninitialized yet!"
                # "If webcam is on, start recording"
                # "Reset trial to zero if exceeded total"
                # "If starting from trial zero, clear and habituate, if not, directly to load trial"
                # "Pre-behavior state and statistics adjustments"
                n195 = local read "Session parameters"() -> (w243:T11)
                n196 = Unbundle By Name(w243) -> ("Start trial"=w238:u16, "Habit tr0 (s)"=w226:i32, "Tone repeat (ms)"=w234:i32, "Reward CR"=w225:bool)
                n197 = local read "Session List Hidden"() -> (w236:u8[])
                n198 = Array Size(array=w236) -> (size(s)=w235:i32)
                n199 = Greater Than 0?(x=w226) -> (x > 0?=w229:bool)
                n200 = Greater Or Equal?(x=w238, y=w235) -> (x >= y?=w239:bool)
                n201 = case shown="True" w239 {
                  tunnel: w238 -> [w257 _]
                  tunnel: [w257 u16 0 ("Curr  tr")] -> w237
                  frame False {
                  }
                  frame True {
                  }
                }
                n202 = Equal To 0?(x=w237) -> (x = 0?=w227:bool)
                n203 = And(x=w227, y=w229) -> (x .and. y?=w228:bool)
                n204 = local read "State info"() -> (w233:T9)
                n205 = Unbundle By Name(w233) -> ("Webcam on"=w232:bool)
                n206 = Bundle By Name(cluster=w233, "Curr  tr"=w237, "Curr State"=pp3_CTL_State."1 Habituation", "Prev State"=pp3_CTL_State."0 NULL", "Total trials memo"=w235, "Tone repeat memo (ms)"=w234, "Webcam recording"=w232) -> (w240:T9)
                n207 = case shown="True" w227 {
                  tunnel: w240 -> [w259 w266]
                  tunnel: w226 -> [_ _]
                  tunnel: [w259 w260] -> w231
                  frame False {
                  }
                  frame True {
                    # "Reset time and info only\nif for 0th trial????!!!"
                    n208 = Tick Count (ms)() -> (millisecond timer value=w265:u32)
                    n209 = To Quad Integer(1:w265) -> (0:w264:i64)
                    n210 = Bundle By Name(cluster=w266, "Curr (ms)"=w264, "Cum (ms)"=i64 0) -> (w260:T9)
                    n211 = local read "Session info"() -> (w261:T12)
                    n212 = call "pp2_updateSessionInfoCLEAR.vi"("Session info In"=w261) -> ("Session info Out"=w262:T12)  [unwired: 10 in]
                    n213 = local write "Session info"(w262) -> ()
                  }
                }
                n214 = case shown="True" w228 {
                  tunnel: w231 -> [w245 w252]
                  tunnel: [w246 w251] -> w230
                  tunnel: w226 -> [_ w250]
                  tunnel: w225 -> [w244 w249]
                  frame False {
                    n215 = call "pp3_trial_NextState.vi"("Reward CR"=w244, "New state countdown (ms)"=i64 0, "New State"=pp3_CTL_State."2 (Load Trial)", "State In"=w245) -> ("State Out"=w246:T9)  [unwired: 7 in]
                  }
                  frame True {
                    # "Habituation only if 0th trial and habituation length >0"
                    n216 = To Quad Integer(1:w250) -> (0:w253:i64)
                    n217 = Multiply(x=w253, y=i64 1000) -> (x*y=w254:i64)
                    n218 = call "pp3_trial_NextState.vi"("Reward CR"=w249, "New state countdown (ms)"=w254, "New State"=pp3_CTL_State."1 Habituation", "State In"=w252) -> ("State Out"=w251:T9)  [unwired: 7 in]
                  }
                }
                n219 = local write "State info"(w230) -> ()
              }
              frame #2 {
                w285 = "\t"
                # "Initialize log directory"
                n220 = Get Date/Time In Seconds() -> (seconds since 1Jan1904=w302:timestamp)
                n221 = local read "Session parameters"() -> (w314:T11)
                n222 = Obtain Queue(name (unnamed)="RL Log Queue", element data type="") -> (queue out=w268:refnum<queue>)  [unwired: 3 in, 2 out]
                n223 = Unbundle By Name(w314) -> ("Log File Directory Root"=w301:path, "Subject Name"=w312:string)
                n224 = Format Date/Time String(time format string (%c)="\\%y%m%d\\%H%M%S\\", seconds (now)=w302) -> (date/time string=w313:string)  [unwired: 1 in]
                n225 = Format Date/Time String(time format string (%c)="%y%m%d_%H%M%S.pp2tt.tsv" ("pattern (all files)"), seconds (now)=w302) -> (date/time string=w310:string)  [unwired: 1 in]
                n226 = Format Date/Time String(time format string (%c)="%y%m%d_%H%M%S.pp2sl.tsv" ("pattern (all files)"), seconds (now)=w302) -> (date/time string=w304:string)  [unwired: 1 in]
                n227 = Format Date/Time String(time format string (%c)="%y%m%d_%H%M%S.pp2rl.tsv" ("pattern (all files)"), seconds (now)=w302) -> (date/time string=w300:string)  [unwired: 1 in]
                n228 = Open VI Reference(type specifier VI Refnum (for type only)=refnum<vi> refnum, vi path=path "C:/Packages/pyonpyon/LV2/impl/pp2_log_SpawnRLLogger.vi", options=128) -> (vi reference=w273:refnum<vi>, error out=w272:errorcluster)  [unwired: 3 in]
                n229 = Concatenate Strings(w312, w313) -> (w311:string)
                n230 = Build Path(base path=w301, name or relative path=w311) -> (appended path=w293:path)
                n231 = Create Folder(path (use dialog)=w293) -> (created path=w287:path)  [unwired: 2 in, 2 out]
                n232 = disable-structure shown="Disabled" {
                  disable-tunnel: w310 -> [w318 _]
                  disable-tunnel: w287 -> [w315 _]
                  frame Disabled {
                    (unwired) TRUE ("Actually Run?")
                    n233 = Build Path(base path=w315, name or relative path=w318) -> (appended path=w317:path)
                    n234 = local read "Trial Types"() -> (w316:T1[])
                    n235 = call "pp3_log_trialTypes.vi"("Trial Types File Path"=w317, "Trial Types"=w316) -> ()  [unwired: 10 in]
                  }
                  frame Enabled {
                  }
                }
                n236 = Build Path(base path=w287, name or relative path=w300) -> (appended path=w269:path)
                n237 = call-by-ref "Start Asynchronous Call"(reference=w273, error in=w272, "file path in"=w269, "queue in"=w268) -> ()  [unwired: 10 in, 2 out]
                n238 = Build Path(base path=w287, name or relative path=w304) -> (appended path=w295:path)
                n239 = local read "Session List Hidden"() -> (w306:u8[])
                n240 = Bundle By Name(cluster=w314, "Log File Directory"=w287) -> (w267:T11)
                n241 = Build Path(base path=w287, name or relative path="cam\\") -> (appended path=w291:path)
                n242 = local read "Info VI Name"() -> (w283:string)
                n243 = local read "Info Hostname"() -> (w284:string)
                n244 = local read "Info VI Revision"() -> (w282:string)
                n245 = Create Folder(path (use dialog)=w291) -> ()  [unwired: 2 in, 3 out]
                n246 = local read "Daq config"() -> (w309:T4)
                n247 = call "pp2_log_toString_sessionList.vi"("Session List in"=w306) -> ("spreadsheet string"=w305:string)  [unwired: 10 in]
                n248 = Open/Create/Replace File(file path (use dialog)=w295, operation (0:open)=T14."create") -> (refnum out=w296:refnum<file>)  [unwired: 4 in, 2 out]
                n249 = call "pp2_log_DAQconfig.vi"("queue in"=w268, "Daq config"=w309) -> ("queue out"=w280:refnum<queue>)  [unwired: 9 in]
                n250 = Concatenate Strings("RUNLOG" ("string"), w285, w284, w285, w283, w285, w282, "\r") -> (w278:string)
                n251 = call "pp3_log_sessionParameters.vi"("queue in"=w280, "Session parameters"=w267) -> ("queue out"=w289:refnum<queue>)  [unwired: 9 in]
                n252 = local write "Session parameters"(w267) -> ()
                n253 = Write to Text File(file (use dialog)=w296, text=w305) -> (refnum out=w307:refnum<file>, error out=w308:errorcluster)  [unwired: 2 in, 1 out]
                n254 = call "pp3_log_trialMemo.vi"("queue in"=w289) -> ("queue out"=w290:refnum<queue>)  [unwired: 10 in]
                n255 = Close File(refnum=w307, error in=w308) -> ()  [unwired: 2 out]
                n256 = call "pp3_log_state.vi"("Log memo?"=TRUE, "queue in"=w290) -> ("queue out"=w279:refnum<queue>)  [unwired: 9 in]
                n257 = Enqueue Element(queue=w279, element=w278) -> (queue out=w277:refnum<queue>)  [unwired: 2 in, 2 out]
              }
              frame #3 {
                w330 = 1000 ("y")
                # "Stop whole VI if \"Stop\" pushed or end reached"
                # "Main Behavior Loop"
                n258 = local read "Session parameters"() -> (w349:T11)
                n259 = Unbundle By Name(w349) -> ("ITI max\n(s)"=w337:i32, "ITI min\n(s)"=w336:i32, "Stay \n(s)"=w350:i32, "Jump time\n(s)"=w345:i32, "Shock \ndur (s)"=w344:i32, "Pre click \n(V)"=w341:dbl, "Click\ndel (s)"=w329:dbl, "Reward CR"=w319:bool)
                n260 = local read "Session info"() -> (w323:T12)
                n261 = local read "Runtime Errors"() -> (w332:errorcluster)
                n262 = local read "Daq config"() -> (w331:T4)
                n263 = local read "State info"() -> (w324:T9)
                n264 = Multiply(x=w330, y=w337) -> (x*y=w339:i32)
                n265 = Multiply(x=w330, y=w336) -> (x*y=w338:i32)
                n266 = Multiply(x=w350, y=w330) -> (x*y=w351:i32)
                n267 = Multiply(x=w345, y=w330) -> (x*y=w347:i32)
                n268 = Multiply(x=w344, y=w330) -> (x*y=w346:i32)
                n269 = Multiply(x=w329, y=w330) -> (x*y=w328:dbl)
                n270 = To Quad Integer(1:w338) -> (0:w334:i64)
                n271 = To Quad Integer(1:w347) -> (0:w343:i64)
                n272 = To Quad Integer(1:w339) -> (0:w335:i64)
                n273 = To Quad Integer(1:w351) -> (0:w348:i64)
                n274 = To Quad Integer(1:w346) -> (0:w342:i64)
                n275 = To Quad Integer(1:w328) -> (0:w327:i64)
                n276 = while {
                  shift-right: [w382] -> w326
                  shift-left: w324 -> [w381]
                  shift-right: [w378] -> _
                  shift-left: w323 -> [w386]
                  shift-right: [w379] -> w325
                  shift-left: w331 -> [w385]
                  shift-right: [w362] -> w320
                  shift-left: w322 -> [w356]
                  tunnel: w348 -> [w377]
                  tunnel: w343 -> [w376]
                  tunnel: w342 -> [w375]
                  tunnel: w341 -> [w374]
                  shift-right: [w373] -> w333
                  shift-left: w332 -> [w366]
                  shift-right: [w371] -> _
                  shift-left: FALSE -> [w372]
                  tunnel: w335 -> [w370]
                  tunnel: w334 -> [w369]
                  tunnel: w327 -> [w363]
                  tunnel: [w359] -> w321
                  tunnel: w319 -> [w352]
                  stop <- w365 stop-if-true
                  # "Update error display here"
                  # "Pre click (V)"
                  # "Click del (ms)"
                  # "Jump time (ms)"
                  # "Stay (ms)"
                  # "ITI max/min (ms)"
                  # "Shock dur (ms)"
                  # "Done and timed out"
                  # "Exitable?"
                  # "Once marker\n(reset to False automatically\nat loop end for most types)"
                  # "State timeout?"
                  # "Side changed?"
                  n277 = call "pp3_updateSideState.vi"("error in (no error)"=w366, "log queue in"=w356, "Daq config In"=w385, "State In"=w381) -> ("error out"=w367:errorcluster, "log queue out"=w355:refnum<queue>, "Daq config Out"=w380:T4, "State Out"=w353:T9, "State timeout"=w384:bool, "vid display"=w354:bool, "Side change"=w383:bool)  [unwired: 1 in]
                  n278 = local write "Runtime Errors"(w366) -> ()
                  n279 = case shown="True" w354 {
                    tunnel: w353 -> [_ w387]
                    frame False {
                    }
                    frame True {
                      n280 = local write "State info"(w387) -> ()
                    }
                  }
                  n281 = Unbundle By Name(w353) -> ("Curr State"=w364:T10)
                  n282 = case shown="\"4 Load Audio/Click Delay\"" w364 {
                    selector: w364 -> [_ _ _ _ w516 _ _ _ _]
                    tunnel: w386 -> [w396 w418 w438 w488 w524 w589 w619 w639 w691]
                    tunnel: w353 -> [w399 w410 w442 w477 w528 w593 w623 w640 w690]
                    tunnel: w384 -> [w390 _ w439 w486 w526 w592 _ w644 w687]
                    tunnel: w383 -> [_ _ w443 _ w529 w591 _ _ _]
                    tunnel: [w398 w424 w441 w489 w527 w596 w622 w643 w690] -> w382
                    tunnel: w380 -> [w397 w422 w437 w481 w522 w585 w615 w635 w689]
                    tunnel: [w397 w421 w434 w480 w521 w584 w615 w632 w689] -> w379
                    tunnel: [w396 w418 w438 w488 w524 w589 w619 w638 w691] -> w378
                    tunnel: w377 -> [_ w419 w440 _ _ _ _ _ _]
                    tunnel: w376 -> [_ _ _ w490 _ _ _ _ _]
                    tunnel: w375 -> [_ _ _ _ w525 _ _ _ _]
                    tunnel: w374 -> [_ _ w431 _ _ _ _ _ _]
                    tunnel: w367 -> [w394 w417 w436 w482 w520 w583 w618 w634 w692]
                    tunnel: [w394 w416 w435 w479 w519 w582 w618 w633 w692] -> w373
                    tunnel: w372 -> [_ _ _ w484 _ _ _ w642 w693]
                    tunnel: [FALSE FALSE FALSE w483 FALSE FALSE FALSE w641 w693] -> w371
                    tunnel: w370 -> [_ _ _ _ _ w595 w625 _ _]
                    tunnel: w369 -> [_ _ _ _ _ w594 w624 _ _]
                    tunnel: [TRUE FALSE FALSE FALSE FALSE FALSE FALSE TRUE TRUE] -> w368
                    tunnel: w363 -> [_ _ w430 _ _ _ _ _ _]
                    tunnel: w355 -> [w391 w408 w429 w485 w517 w587 w616 w636 w688]
                    tunnel: [w391 w407 w429 w485 w517 w587 w616 w636 w688] -> w362
                    tunnel: [FALSE ("State timeout") FALSE ("State timeout") FALSE ("State timeout") FALSE ("State timeout") FALSE ("State timeout") FALSE ("State timeout") FALSE ("State timeout") FALSE ("State timeout") w687] -> w357
                    tunnel: w352 -> [w388 w406 w426 w474 w513 w580 w613 w628 _]
                    frame "1 Habituation" {
                      n283 = case shown="True" w390 {
                        tunnel: w399 -> [w400 w405]
                        tunnel: [w400 w404] -> w398
                        tunnel: w388 -> [_ w401]
                        frame False {
                        }
                        frame True {
                          # "Load next if timeout"
                          n284 = call "pp3_trial_NextState.vi"("Reward CR"=w401, "New state countdown (ms)"=i64 0, "New State"=pp3_CTL_State."2 (Load Trial)", "State In"=w405) -> ("State Out"=w404:T9)  [unwired: 7 in]
                        }
                      }
                      n285 = Wait Until Next ms Multiple(millisecond multiple=u32 3) -> ()  [unwired: 1 out]
                    }
                    frame "2 (Load Trial)" {
                      # "Load curr trial and apply variable shock if on.\n(will not increment)"
                      n286 = local read "Session param (dynamic)"() -> (w413:T8)
                      n287 = local read "Session List Hidden"() -> (w414:u8[])
                      n288 = disable-structure shown="Disabled" {
                        frame Disabled {
                          n289 = Wait Until Next ms Multiple(millisecond multiple=u32 1) -> ()  [unwired: 1 out]
                        }
                        frame Enabled {
                        }
                      }
                      n290 = local read "Trial Types"() -> (w415:T1[])
                      n291 = call "pp3_trial_loadNext.vi"("State Info In"=w410, "Session param (dynamic)"=w413, "Session List (Hidden variable)"=w414, "Trial Types"=w415, "Daq config In"=w422, "log queue in"=w408, "error in (no error)"=w417) -> ("State Info Out"=w423:T9, "Daq config Out"=w421:T4, "log queue out"=w407:refnum<queue>, "error out"=w416:errorcluster)  [unwired: 5 in]
                      n292 = call "pp3_trial_NextState.vi"("Reward CR"=w406, "New state countdown (ms)"=w419, "New State"=pp3_CTL_State."3 Stay Period", "State In"=w423) -> ("State Out"=w424:T9)  [unwired: 7 in]
                    }
                    frame "3 Stay Period" {
                      n293 = case shown="False" w443 {
                        tunnel: w442 -> [w453 w473]
                        tunnel: [w447 w472] -> w441
                        tunnel: w440 -> [_ w470]
                        tunnel: w439 -> [w452 _]
                        tunnel: w437 -> [w451 w469]
                        tunnel: w436 -> [w450 w468]
                        tunnel: [w449 w468] -> w435
                        tunnel: [w448 w469] -> w434
                        tunnel: w431 -> [w446 _]
                        tunnel: w430 -> [w445 _]
                        tunnel: w426 -> [w444 w467]
                        frame False {
                          n294 = case shown="True" w452 {
                            tunnel: w453 -> [w456 w466]
                            tunnel: w451 -> [w455 w464]
                            tunnel: w450 -> [w454 w463]
                            tunnel: [w454 w462] -> w449
                            tunnel: [w455 w461] -> w448
                            tunnel: [w456 w460] -> w447
                            tunnel: w446 -> [_ w459]
                            tunnel: w445 -> [_ w458]
                            tunnel: w444 -> [_ w457]
                            frame False {
                              # "No side change, no timeout"
                            }
                            frame True {
                              # "If stay timed out without side change, \ntrigger change to (Load audio) and play click"
                              n295 = call "pp3_trial_NextState.vi"("Reward CR"=w457, "New state countdown (ms)"=w458, "New State"=pp3_CTL_State."4 Load Audio/Click Delay", "State In"=w466) -> ("State Out"=w460:T9)  [unwired: 7 in]
                              n296 = call "pp3_DAQ_AudioClick.vi"("State In"=w460, "Daq config"=w464, "Pre click \n(V)"=w459, "error in (no error)"=w463) -> ("Daq config 2"=w461:T4, "error out"=w462:errorcluster)  [unwired: 5 in]
                            }
                          }
                        }
                        frame True {
                          # "If side changed during stay, reload stay period\n(will not log state change, 3 == 3)"
                          n297 = call "pp3_trial_NextState.vi"("Reward CR"=w467, "New state countdown (ms)"=w470, "New State"=pp3_CTL_State."3 Stay Period", "State In"=w473) -> ("State Out"=w472:T9)  [unwired: 7 in]
                        }
                      }
                      n298 = Wait Until Next ms Multiple(millisecond multiple=u32 3) -> ()  [unwired: 1 out]
                    }
                    frame "4 Load Audio/Click Delay" {
                      n299 = case shown="False" w484 {
                        selector: w484 -> [_ w500]
                        tunnel: [TRUE w500] -> w483
                        tunnel: w482 -> [w497 w501]
                        tunnel: w481 -> [w496 w502]
                        tunnel: [w495 w502] -> w480
                        tunnel: [w494 w501] -> w479
                        tunnel: w477 -> [w493 w499]
                        tunnel: [w491 w499] -> w476
                        frame False {
                          # "Load audio just once"
                          n300 = call "pp3_DAQ_AudioLoadStimulus.vi"("State Info In"=w493, "Daq config In"=w496, "error in (no error)"=w497) -> ("Daq config Out"=w495:T4, "error out"=w494:errorcluster)  [unwired: 11 in]
                          n301 = Bundle By Name(cluster=w493, "Tone countdown (ms)"=i64 0) -> (w491:T9)
                        }
                        frame True {
                        }
                      }
                      n302 = case shown="True" w486 {
                        tunnel: w490 -> [_ w507]
                        tunnel: [w503 w508] -> w489
                        tunnel: w476 -> [w503 w505]
                        tunnel: w474 -> [_ w504]
                        frame False {
                        }
                        frame True {
                          n303 = Unbundle By Name(w505) -> ("Current Loaded Trial.Trial Type"=w509:T2)
                          n304 = case shown="\"TEST\", Default" w509 {
                            tunnel: [pp3_CTL_State."5 GO Trial" ("New State") pp3_CTL_State."11 TEST Trial" ("New State") pp3_CTL_State."8 NOGO Trial" ("New State")] -> w506
                            frame "GO" {
                            }
                            frame "TEST", Default {
                            }
                            frame "NOGO" {
                            }
                          }
                          n305 = call "pp3_trial_NextState.vi"("Reward CR"=w504, "New state countdown (ms)"=w507, "New State"=w506, "State In"=w505) -> ("State Out"=w508:T9)  [unwired: 7 in]
                        }
                      }
                      n306 = Wait Until Next ms Multiple(millisecond multiple=u32 3) -> ()  [unwired: 1 out]
                    }
                    frame "5 GO Trial", "8 NOGO Trial", "11 TEST Trial" {
                      n307 = case shown="False" w529 {
                        tunnel: w528 -> [w538 w568]
                        tunnel: [w537 w571] -> w527
                        tunnel: w526 -> [w539 _]
                        tunnel: w525 -> [w536 w564]
                        tunnel: w522 -> [w535 w569]
                        tunnel: [w534 w569] -> w521
                        tunnel: w520 -> [w533 w570]
                        tunnel: [w532 w570] -> w519
                        tunnel: w516 -> [w531 w567]
                        tunnel: w513 -> [w530 w563]
                        frame False {
                          n308 = case shown="True" w539 {
                            tunnel: w538 -> [w541 w554]
                            tunnel: [w540 w553] -> w537
                            tunnel: w536 -> [_ w548]
                            tunnel: w535 -> [w545 w551]
                            tunnel: [w544 w551] -> w534
                            tunnel: w533 -> [w543 w552]
                            tunnel: [w542 w552] -> w532
                            tunnel: w531 -> [_ w547]
                            tunnel: w530 -> [_ w546]
                            frame False {
                              # "continue/start  sound,\nretrigger if necessary"
                              n309 = call "pp3_DAQ_AudioTriggerPlay.vi"("Daq config In"=w545, "State In"=w541, "error in (no error)"=w543) -> ("Daq config Out"=w544:T4, "State Out"=w540:T9, "error out"=w542:errorcluster)  [unwired: 10 in]
                            }
                            frame True {
                              n310 = case shown="\"5 GO Trial\"" w547 {
                                selector: w547 -> [w556 _ _ _]
                                tunnel: [w556 pp3_CTL_State."7 GO Timeout" ("New State") pp3_CTL_State."10 NOGO Timeout" ("New State") pp3_CTL_State."13 TEST Timeout" ("New State")] -> w550
                                tunnel: [i64 0 ("New state countdown (ms)") w557 i64 0 ("New state countdown (ms)") i64 0 ("New state countdown (ms)")] -> w549
                                tunnel: w548 -> [_ w557 _ _]
                                frame Default {
                                # "Will not happen"
                                }
                                frame "5 GO Trial" {
                                # "If timout, miss!!!"
                                }
                                frame "8 NOGO Trial" {
                                # "If time out,\ncorrect rejection!!!"
                                }
                                frame "11 TEST Trial" {
                                }
                              }
                              n311 = call "pp3_trial_NextState.vi"("Reward CR"=w546, "New state countdown (ms)"=w549, "New State"=w550, "State In"=w554) -> ("State Out"=w553:T9)  [unwired: 7 in]
                            }
                          }
                        }
                        frame True {
                          n312 = case shown="\"5 GO Trial\"" w567 {
                            selector: w567 -> [w573 _ _ _]
                            tunnel: [w573 pp3_CTL_State."6 GO Jumped" ("New State") pp3_CTL_State."9 NOGO Jumped" ("New State") pp3_CTL_State."12 TEST Jumped" ("New State")] -> w565
                            tunnel: [i64 0 ("New state countdown (ms)") i64 0 ("New state countdown (ms)") w576 i64 0 ("New state countdown (ms)")] -> w566
                            tunnel: w564 -> [_ _ w576 _]
                            frame Default {
                              # "Will not happen"
                            }
                            frame "5 GO Trial" {
                              # "If side changed, hit!!!"
                            }
                            frame "8 NOGO Trial" {
                              # "If side changed,\nfalse alarm!!!"
                            }
                            frame "11 TEST Trial" {
                              # "If side changed, hit!!!"
                            }
                          }
                          n313 = call "pp3_trial_NextState.vi"("Reward CR"=w563, "New state countdown (ms)"=w566, "New State"=w565, "State In"=w568) -> ("State Out"=w571:T9)  [unwired: 7 in]
                        }
                      }
                      n314 = Wait Until Next ms Multiple(millisecond multiple=u32 3) -> ()  [unwired: 1 out]
                    }
                    frame "7 GO Timeout", "9 NOGO Jumped" {
                      # "Shock end should be ASAP"
                      n315 = Or(x=w591, y=w592) -> (x .or. y?=w590:bool)
                      n316 = case shown="True" w590 {
                        tunnel: [w598 w611] -> w596
                        tunnel: w595 -> [_ w610]
                        tunnel: w594 -> [_ w609]
                        tunnel: w593 -> [w599 w607]
                        tunnel: w585 -> [w603 w606]
                        tunnel: [w602 w606] -> w584
                        tunnel: w583 -> [w601 w605]
                        tunnel: [w600 w605] -> w582
                        tunnel: w580 -> [_ w604]
                        frame False {
                          # "continue/start  sound,\nretrigger if necessary"
                          # "Continue shock"
                          n317 = call "pp3_DAQ_AudioTriggerPlay.vi"("Daq config In"=w603, "State In"=w599, "error in (no error)"=w601) -> ("Daq config Out"=w602:T4, "State Out"=w598:T9, "error out"=w600:errorcluster)  [unwired: 10 in]
                        }
                        frame True {
                          # "If side change or timeout,\nnext state (end shock)"
                          n318 = call "RandomInt64.vi"("Min"=w609, "Max"=w610) -> ("Random"=w608:i64)  [unwired: 9 in]
                          n319 = call "pp3_trial_NextState.vi"("Reward CR"=w604, "New state countdown (ms)"=w608, "New State"=pp3_CTL_State."14 Intertrial Interval", "State In"=w607) -> ("State Out"=w611:T9)  [unwired: 7 in]
                        }
                      }
                      n320 = Wait Until Next ms Multiple(millisecond multiple=u32 1) -> ()  [unwired: 1 out]
                    }
                    frame "6 GO Jumped", "10 NOGO Timeout", "12 TEST Jumped", "13 TEST Timeout" {
                      # "Response correct,\ngo to ITI immediately"
                      n321 = disable-structure shown="Disabled" {
                        frame Disabled {
                          n322 = Wait Until Next ms Multiple(millisecond multiple=u32 1) -> ()  [unwired: 1 out]
                        }
                        frame Enabled {
                        }
                      }
                      n323 = call "RandomInt64.vi"("Min"=w624, "Max"=w625) -> ("Random"=w621:i64)  [unwired: 9 in]
                      n324 = call "pp3_trial_NextState.vi"("Reward CR"=w613, "New state countdown (ms)"=w621, "New State"=pp3_CTL_State."14 Intertrial Interval", "State In"=w623) -> ("State Out"=w622:T9)  [unwired: 7 in]
                    }
                    frame "14 Intertrial Interval" {
                      n325 = case shown="False" w642 {
                        selector: w642 -> [_ w670]
                        tunnel: [TRUE w670] -> w641
                        tunnel: w640 -> [w648 w666]
                        tunnel: w639 -> [w659 w669]
                        tunnel: [w656 w669] -> w638
                        tunnel: w635 -> [w654 w668]
                        tunnel: w634 -> [w653 w667]
                        tunnel: [w657 w667] -> w633
                        tunnel: [w658 w668] -> w632
                        tunnel: [w655 w666] -> w629
                        frame False {
                          # "Paint done trial in table"
                          # "Runs just first cycle!"
                          # "Update stats/close audio"
                          n326 = call "pp3_updateSessionInfo.vi"("Session info In"=w659, "State In"=w648) -> ("Session info Out"=w656:T12)  [unwired: 9 in]
                          n327 = Unbundle By Name(w648) -> ("Curr  tr"=w646:u16, "Prev State"=w649:T10)
                          n328 = local write "Session info"(w656) -> ()
                          n329 = call "pp3_DAQ_AudioWaitStop.vi"("State info"=w648, "Daq config In"=w654, "error in (no error)"=w653) -> ("State info out"=w650:T9, "Daq config Out"=w658:T4, "error out"=w657:errorcluster)  [unwired: 10 in]
                          n330 = case shown="\"9 NOGO Jumped\"" w649 {
                            tunnel: [u32 52736 u32 11206570 u32 16731983 u32 16763594 u32 12369084] -> w647
                            frame "6 GO Jumped" {
                            }
                            frame "7 GO Timeout" {
                            }
                            frame "9 NOGO Jumped" {
                            }
                            frame "10 NOGO Timeout" {
                            }
                            frame Default {
                            }
                          }
                          n331 = Bundle By Name(cluster=w650, "Tone\nGate"=FALSE ("Tone\nGate"), "State update flag"=TRUE) -> (w655:T9)
                          n332 = control-ref of="Session list display"() -> (w645:refnum<vi>)
                          n333 = call "pp2_util_paintTableElement.vi"("Color Box"=w647, "Numeric"=w646, "Tbl Refnum"=w645) -> ()  [unwired: 9 in]
                        }
                        frame True {
                        }
                      }
                      n334 = Wait Until Next ms Multiple(millisecond multiple=u32 3) -> ()  [unwired: 1 out]
                      n335 = case shown="True" w644 {
                        tunnel: [w671 w679] -> w643
                        tunnel: w629 -> [w671 w673]
                        tunnel: w628 -> [_ w672]
                        frame False {
                        }
                        frame True {
                          # "Exit if last trial fin\n15s extra video"
                          n336 = Unbundle By Name(w673) -> ("Curr  tr"=w681:u16, "Total trials memo"=w677:i64)
                          n337 = Increment(x=w681) -> (x+1=w675:u16)
                          n338 = Greater Or Equal?(x=w675, y=w677) -> (x >= y?=w676:bool)
                          n339 = case shown="False" w676 {
                            tunnel: [pp3_CTL_State."15 Done" ("New State") pp3_CTL_State."2 (Load Trial)" ("New State")] -> w678
                            tunnel: [i64 15000 ("New state countdown (ms)") i64 0 ("New state countdown (ms)")] -> w674
                            frame True {
                            }
                            frame False {
                            }
                          }
                          n340 = Bundle By Name(cluster=w673, "Curr  tr"=w675) -> (w680:T9)
                          n341 = call "pp3_trial_NextState.vi"("Reward CR"=w672, "New state countdown (ms)"=w674, "New State"=w678, "State In"=w680) -> ("State Out"=w679:T9)  [unwired: 7 in]
                        }
                      }
                    }
                    frame "0 NULL", "15 Done" {
                      # "When \"15 Done\" times out,\nsignal will be sent to exit the \nloop"
                      # "\"0 Null\" Will not happen, added to fix compile error"
                      n342 = Wait Until Next ms Multiple(millisecond multiple=u32 3) -> ()  [unwired: 1 out]
                    }
                  }
                  n343 = local read "stop"() -> (w361:bool)
                  n344 = Or(x=w361, y=w357) -> (x .or. y?=w359:bool)
                  n345 = Or(x="Pause", y=w359) -> (x .or. y?=w358:bool)
                  n346 = And(x=w368, y=w358) -> (x .and. y?=w365:bool)
                }
                n347 = local write "Daq config"(w325) -> ()
                n348 = local write "State info"(w326) -> ()
              }
              frame #4 {
                # "Will close log file"
                n349 = flat-sequence {
                  frame #0 {
                    # "This done in \"15 Done\"\nloop instead"
                    n350 = disable-structure shown="Disabled" {
                      frame Disabled {
                        # "Always record at least\n10 extra seconds of video"
                        n351 = Wait (ms)(milliseconds to wait=u32 10000) -> ()  [unwired: 1 out]
                      }
                      frame Enabled {
                      }
                    }
                  }
                  frame #1 {
                    w700 = FALSE
                    # "This will stop webcam recording in\nasynchronous processs"
                    n352 = local read "State info"() -> (w701:T9)
                    n353 = Bundle By Name(cluster=w701, "Tone\nGate"=w700, "Punish"=w700, "Current DAQ DO Int"=u16 0, "Webcam recording"=w700) -> (w702:T9)
                    n354 = local write "State info"(w702) -> ()
                  }
                }
                n355 = Release Queue(queue=w695, error in (no error)=w696) -> (error out=w697:errorcluster)  [unwired: 1 in, 2 out]
                n356 = local write "Runtime Errors"(w697) -> ()
              }
              frame #5 {
                # "Post-behavior UI adjustments"
                n357 = local read "Runtime Errors"() -> (w704:errorcluster)
                n358 = local read "Daq config"() -> (w706:T4)
                n359 = property on="Pause" class="Bool (strict)"("DisabledEnum"=T13."Disabled and Grayed Out" ("Disabled")) -> ()  [unwired: 2 in, 2 out]
                n360 = property on="Trial Types Control" class="TabCtl (strict)"("DisabledEnum"=T13."Enabled" ("Disabled")) -> ()  [unwired: 2 in, 2 out]
                n361 = call "pp2_DAQwriteDO.vi"("error in (no error)"=w704, "Daq config"=w706, "DAQ Digital In"=u16 0) -> ("error out"=w703:errorcluster, "Daq config 2"=w707:T4)  [unwired: 7 in]
                n362 = local write "Daq config"(w707) -> ()
                n363 = local write "Runtime Errors"(w703) -> ()
              }
            }
          }
        }
      }
    }
    frame #4 {
      w719 = FALSE ("Webcam on")
      w722 = FALSE
      w718 = T13."Enabled" ("Disabled")
      # "Close task only if video used"
      # "Clean up DAQ"
      # "Stop webcam recording"
      # "Post UI Adjustments"
      n364 = local read "State info"() -> (w720:T9)
      n365 = Bundle By Name(cluster=w720, "Webcam on"=w719, "Webcam recording"=w719) -> (w721:T9)
      n366 = local write "State info"(w721) -> ()
      n367 = property on="Daq config" class="Clust (strict)"("DisabledEnum"=w718) -> ()  [unwired: 2 in, 2 out]
      n368 = property on="Session List Control" class="TabCtl (strict)"("DisabledEnum"=w718) -> ()  [unwired: 2 in, 2 out]
      n369 = property on="Trial Types Control" class="TabCtl (strict)"("DisabledEnum"=w718) -> ()  [unwired: 2 in, 2 out]
      n370 = property on="Session param (dynamic)" class="Clust (strict)"("DisabledEnum"=w718) -> ()  [unwired: 2 in, 2 out]
      n371 = property on="State info" class="Clust (strict)"("DisabledEnum"=w718) -> ()  [unwired: 2 in, 2 out]
      n372 = property on="Session parameters" class="Clust (strict)"("DisabledEnum"=w718) -> ()  [unwired: 2 in, 2 out]
      n373 = property on="Session info" class="Clust (strict)"("DisabledEnum"=w718) -> ()  [unwired: 2 in, 2 out]
      n374 = property on="Session list display" class="Tbl (strict)"("Visible"=TRUE) -> ()  [unwired: 2 in, 2 out]
      n375 = local read "Runtime Errors"() -> (w715:errorcluster)
      n376 = local read "Daq config"() -> (w716:T4)
      n377 = local write "stop"(w722) -> ()
      n378 = local write "Pause"(w722) -> ()
      n379 = call "pp2_DAQclear.vi"("error in (no error)"=w715, "Daq config in"=w716) -> ("error out"=w712:errorcluster, "Daq config out"=w717:T4)  [unwired: 8 in]
      n380 = local write "Daq config"(w717) -> ()
      n381 = case shown="True" w711 {
        tunnel: w714 -> [_ w726]
        tunnel: [w723 w725] -> w713
        tunnel: w712 -> [w723 w724]
        frame False {
        }
        frame True {
          n382 = Close Reference(reference=w726, error in (no error)=w724) -> (error out=w725:errorcluster)
        }
      }
      n383 = local write "Runtime Errors"(w713) -> ()
    }
    frame #5 {
      # "Take screenshot for records"
      n384 = local read "Session parameters"() -> (w733:T11)
      n385 = Unbundle By Name(w733) -> ("Log File Directory"=w734:path)
      n386 = control-ref of="This VI"() -> (w730:refnum<vi>)
      n387 = Format Date/Time String(time format string (%c)="%y%m%d_%H%M%S.pp2ss.png" ("pattern (all files)")) -> (date/time string=w731:string)  [unwired: 2 in]
      n388 = Build Path(base path=w734, name or relative path=w731) -> (appended path=w727:path)
      n389 = invoke class="VI" method="FP.Get Image"(reference=w730, "image depth"=24 ("Image Depth")) -> ("image data"=w728:T15)  [unwired: 4 in, 5 out]
      n390 = call <vilib>:"Write PNG File.vi"("image data"=w728, "path to PNG file"=w727) -> ()  [unwired: 8 in, 2 out]
    }
  }
